vi "single fit V5.vi"(0 "single fit parameters":T11={"number of 2D grid points"=300, "# of points in pond"=339, "# of points in window"=10919, "decimation threshold"=1, "normalization factor"=0.029014793, "pond scale factor "=3.0, "normalized z"=[], "decimated z"=[], "decimated omega"=[], "omega in window"=[], "z in window"=[], "data center"=3.0+0.0i, "inverse"=[], "linear "=[], "omega around"=[], "phase around center"=[], "fit for phase around senter "=[], "three points"={[], []}, "max omega"=0.029014793, "min omega"=0.029014793, "dz/domega"=[]}, 1 "plot what":enum16{"plot", "dont plot", "a"}(ring), 2 "find fit action":T8=enum."bbb", 3 "cursor bracket: fragment  ref":refnum<vi>, 5 "omega map parameters":T10={"map method"=enum."less trivial", "2:window factor"=1, "left"=3.0, "right"=3.0, "omega"=3.0, "gamma"=3.0, "theta0"=3.0, "use points"=enum."decimated", "z(inf) method"=enum."median"}, 7 "parameters: wavepacket":T4={"R"=0.5, "wave number"=9.317073170731707, "delta k"=8.0, "radii vector"=[-1.5, -1.4361702127659575, -1.372340425531915, -1.3085106382978724, -1.2446808510638299, -1.1808510638297873, -1.1170212765957448, -1.0531914893617023, -0.9893617021276596, -0.9255319148936171, -0.8617021276595745, -0.797872340425532, -0.7340425531914894, -0.6702127659574468, -0.6063829787234043, -0.5425531914893618, -0.47872340425531923, -0.4148936170212767, -0.35106382978723416, -0.2872340425531916, -0.2234042553191491, -0.15957446808510656, -0.09574468085106402, -0.03191489361702149, 0.03191489361702127, 0.0957446808510638, 0.15957446808510634, 0.22340425531914887, 0.2872340425531914, 0.35106382978723394, 0.4148936170212765, 0.478723404255319, 0.5425531914893615, 0.6063829787234041, 0.6702127659574466, 0.7340425531914891, 0.7978723404255317, 0.8617021276595742, 0.9255319148936167, 0.9893617021276593, 1.0531914893617018, 1.1170212765957444, 1.1808510638297869, 1.2446808510638294, 1.308510638297872, 1.3723404255319145, 1.436170212765957], "radial section"=[-0.0004435445083409722-0.0006849119769038184i, -0.0019041504025470312+0.00048506615579312746i, -0.00033819317362592454+0.00445256884703147i, 0.008816469374270853+0.0037385059601190047i, 0.012871051762105094-0.014489928742809924i, -0.018368300887416027-0.03213667871181133i, -0.06546452421830008+0.012862287260149104i, -0.014850036489490822+0.11250194158627941i, 0.16349796399613198+0.08029027224632529i, 0.19438455385148304-0.19581588584379236i, -0.1764517694229995-0.3527505964833319i, -0.5269831636950821+0.07349813170268539i, -0.12571385568454752+0.6656158756342778i, 0.7094879059571741+0.3986438774133789i, 0.6853115356988965-0.6177994674685856i, -0.39205198313530026-0.9060192033187687i, -0.9933425353192824+0.08278273424671147i, -0.22770617853759392+0.9220982637950581i, 0.720265950295077+0.4589746661280373i, 0.564369978321562-0.45471185099562045i, -0.20063123992670956-0.5446207511436068i, -0.438459632746935+0.012155082564416607i, -0.0917074180027409+0.299079584121901i, 0.17101533661135507+0.12280738192151135i, 0.17101533661135532+0.1228073819215104i, -0.0917074180027395+0.299079584121901i, -0.4384596327469345+0.01215508256441854i, -0.2006312399267118-0.5446207511436055i, 0.5643699783215596-0.4547118509956226i, 0.7202659502950789+0.45897466612803384i, -0.22770617853759056+0.9220982637950585i, -0.9933425353192818+0.08278273424671675i, -0.3920519831353035-0.9060192033187675i, 0.6853115356988935-0.6177994674685894i, 0.7094879059571758+0.3986438774133766i, -0.12571385568454407+0.665615875634279i, -0.5269831636950825+0.0734981317026883i, -0.17645176942300106-0.3527505964833319i, 0.19438455385148207-0.19581588584379414i, 0.16349796399613292+0.0802902722463243i, -0.014850036489490074+0.11250194158627992i, -0.06546452421830022+0.012862287260149614i, -0.018368300887416446-0.032136678711811265i, 0.012871051762104992-0.014489928742810118i, 0.008816469374270927+0.0037385059601189627i, -0.0003381931736258947+0.004452568847031496i, -0.0019041504025470377+0.00048506615579315077i], "wave vector"=19.513632417419526, "wavepacket is"=TRUE} {"delta k" format="%#_3f"; "wave number" format="%#_3f"; "R" format="%#_3f"}, 9 "parameters: complex fit":T3={"main VI path"=path "", "scale factor"=3.0, "# of grid points"=200, "parameters: wavepacket"={"R"=0.5, "wave number"=22.0, "delta k"=7.0, "radii vector"=[], "radial section"=[], "wave vector"=22.0, "wavepacket is"=TRUE}, "span"=0.27789, "interference ?"=enum."cp z center", "filter method"=enum."three"} {"span" min=0.0 max=0.5 step=1e-05 scale=0.0001..0.5 scale format="%#_5f"; "parameters: wavepacket"."delta k" format="%#_3f"; "parameters: wavepacket"."wave number" format="%#_3f"; "parameters: wavepacket"."R" format="%#_3f"}, 11 "input":cdb, 13 "plots: filter related":T6) -> (4 "single fit parameters out":T11={"number of 2D grid points"=300, "# of points in pond"=339, "# of points in window"=10919, "decimation threshold"=1, "normalization factor"=0.029014793, "pond scale factor "=3.0, "normalized z"=[], "decimated z"=[], "decimated omega"=[], "omega in window"=[], "z in window"=[], "data center"=3.0+0.0i, "inverse"=[], "linear "=[], "omega around"=[], "phase around center"=[], "fit for phase around senter "=[], "three points"={[], []}, "max omega"=0.029014793, "min omega"=0.029014793, "dz/domega"=[]}, 6 "omega map parameters out":T10={"map method"=enum."less trivial", "2:window factor"=1, "left"=3.0, "right"=3.0, "omega"=3.0, "gamma"=3.0, "theta0"=3.0, "use points"=enum."decimated", "z(inf) method"=enum."median"}, 8 "parameters: wavepacket  out":T4={"R"=0.5, "wave number"=9.317073170731707, "delta k"=8.0, "radii vector"=[-1.5, -1.4361702127659575, -1.372340425531915, -1.3085106382978724, -1.2446808510638299, -1.1808510638297873, -1.1170212765957448, -1.0531914893617023, -0.9893617021276596, -0.9255319148936171, -0.8617021276595745, -0.797872340425532, -0.7340425531914894, -0.6702127659574468, -0.6063829787234043, -0.5425531914893618, -0.47872340425531923, -0.4148936170212767, -0.35106382978723416, -0.2872340425531916, -0.2234042553191491, -0.15957446808510656, -0.09574468085106402, -0.03191489361702149, 0.03191489361702127, 0.0957446808510638, 0.15957446808510634, 0.22340425531914887, 0.2872340425531914, 0.35106382978723394, 0.4148936170212765, 0.478723404255319, 0.5425531914893615, 0.6063829787234041, 0.6702127659574466, 0.7340425531914891, 0.7978723404255317, 0.8617021276595742, 0.9255319148936167, 0.9893617021276593, 1.0531914893617018, 1.1170212765957444, 1.1808510638297869, 1.2446808510638294, 1.308510638297872, 1.3723404255319145, 1.436170212765957], "radial section"=[-0.0004435445083409722-0.0006849119769038184i, -0.0019041504025470312+0.00048506615579312746i, -0.00033819317362592454+0.00445256884703147i, 0.008816469374270853+0.0037385059601190047i, 0.012871051762105094-0.014489928742809924i, -0.018368300887416027-0.03213667871181133i, -0.06546452421830008+0.012862287260149104i, -0.014850036489490822+0.11250194158627941i, 0.16349796399613198+0.08029027224632529i, 0.19438455385148304-0.19581588584379236i, -0.1764517694229995-0.3527505964833319i, -0.5269831636950821+0.07349813170268539i, -0.12571385568454752+0.6656158756342778i, 0.7094879059571741+0.3986438774133789i, 0.6853115356988965-0.6177994674685856i, -0.39205198313530026-0.9060192033187687i, -0.9933425353192824+0.08278273424671147i, -0.22770617853759392+0.9220982637950581i, 0.720265950295077+0.4589746661280373i, 0.564369978321562-0.45471185099562045i, -0.20063123992670956-0.5446207511436068i, -0.438459632746935+0.012155082564416607i, -0.0917074180027409+0.299079584121901i, 0.17101533661135507+0.12280738192151135i, 0.17101533661135532+0.1228073819215104i, -0.0917074180027395+0.299079584121901i, -0.4384596327469345+0.01215508256441854i, -0.2006312399267118-0.5446207511436055i, 0.5643699783215596-0.4547118509956226i, 0.7202659502950789+0.45897466612803384i, -0.22770617853759056+0.9220982637950585i, -0.9933425353192818+0.08278273424671675i, -0.3920519831353035-0.9060192033187675i, 0.6853115356988935-0.6177994674685894i, 0.7094879059571758+0.3986438774133766i, -0.12571385568454407+0.665615875634279i, -0.5269831636950825+0.0734981317026883i, -0.17645176942300106-0.3527505964833319i, 0.19438455385148207-0.19581588584379414i, 0.16349796399613292+0.0802902722463243i, -0.014850036489490074+0.11250194158627992i, -0.06546452421830022+0.012862287260149614i, -0.018368300887416446-0.032136678711811265i, 0.012871051762104992-0.014489928742810118i, 0.008816469374270927+0.0037385059601189627i, -0.0003381931736258947+0.004452568847031496i, -0.0019041504025470377+0.00048506615579315077i], "wave vector"=19.513632417419526, "wavepacket is"=TRUE} {"delta k" format="%#_3f"; "wave number" format="%#_3f"; "R" format="%#_3f"}, 14 "complex region out":T7={"max re"=1.1965102077412717, "min re"=-1.8034897922587283, "max im"=1.1920568931854867, "min im"=-1.636084117505164, "delta re"=3.0, "delta im"=2.8281410106906506, "center re"=-0.3034897922587282, "delta  z"=3.0+2.8281410106906506i, "center im"=-0.2220136121598386, "center z"=-0.3034897922587282+2.8281410106906506i, "d im"=0.0, "d re"=0.0, "d z"=0.0+0.0i}, 15 "lorentzian out":T1={"Amplitude"=-1.0311345636926572, "omega(0)"=-1.0311345636926572, "Gamma"=-1.0311345636926572, "phase"=-1.0311345636926572, "Q"=-1.0311345636926572, "Norm  Ampl"=-1.0311345636926572, "z (inf)"=-1.0311345636926572+0.0i, "4corners"={"z (-pi/2)"=-1.0311345636926572+0.5736824521422934i, "z(inf)"=-0.5200164984937075+1.0975277942502903i, "z (pi/2)"=-1.0311345636926572+0.5736824521422934i, "z center"=-0.5136528600391839+0.580046090596817i, "z(0)"=-0.5200164984937075+1.0975277942502903i, "radius"=-1.0311345636926572}} {"z (inf)" format="%#9_9f"; "Q" format="%#9_9f"; "phase" format="%#9_9f"; "Gamma" format="%#9_9f"; "omega(0)" format="%#9_9f"})   [LabVIEW 2015]
uses:
  lorentzian.ctl
  circle corners.ctl
  complex region.ctl
  single fit parameters.ctl
  omega map parameters.ctl
  cursor winow.ctl
  find peak action.ctl
  wavepacket.ctl
  plot refs -- filter related.ctl
  peak -- parameters -- complex fit.ctl
  filter method control.ctl
  stack action -- control.ctl
  cursor window action.ctl
  Q - not nan -- integer.vi
  peak - simple guess at omega.vi
  peak - less simple guess at omega.vi
  peak - fix phase.vi
  peak - fit phase around center - V1.vi
  peak - geometry fit.vi
  find circle corners V3.vi
  peak - phase around center.vi
  peak - linear and inverse maps.vi
  array smart append -- complex.vi
  array smart append -- real.vi
  array - rotate - col.vi
  array - rotate - row.vi
  array -- 2D mean .vi
  tale of three indices.vi
  filter -- window span logic.vi
  linear interp iiii- complex - z-omega - divide.vi
  linear interpolation iiii- complex.vi
  containing bix.vi
  peak -- guess at omega -- dzdomega.vi
  <vilib>/Utility/error.llb/Clear Errors.vi
  <vilib>/Analysis/baseanly.llb/Median.vi
  <vilib>/Analysis/baseanly.llb/Mean.vi
  <vilib>/Analysis/baseanly.llb/Mean (DBL).vi
  <vilib>/Analysis/2dsp.llb/Unwrap Phase.vi
  <vilib>/Analysis/baseanly.llb/A x B.vi
  <vilib>/Analysis/baseanly.llb/Real A x B.vi
  command stack.vi
  tale of three indices -- check state.vi
  linear interp iiii- complex - z-omega.vi
  line -- complex.vi
  peak -- z center from mult phase points.vi
  peak -- estimate for lorentzian.vi
  peak -- fake phase around center.vi
  peak -- four corner circle transformation logic.vi
  <vilib>/Analysis/baseanly.llb/Complex A x B.vi
  circle center from three points.vi
  index from range.vi
  <vilib>/gmath/interp.llb/Interpolate 1D.vi
  peak -- fit function -- arctan.vi
  <vilib>/gmath/NumericalOptimization/Nonlinear Curve Fit.vi
  <vilib>/gmath/NumericalOptimization/Nonlinear Curve Fit LM.vi
  <vilib>/Analysis/6fits.llb/Linear Fit.vi
  <vilib>/Analysis/Matrix/Numeric/Conversions/Array To Matrix.vi
  <vilib>/Analysis/Matrix/Numeric/Conversions/Array To Matrix - CA2.vi
  <vilib>/Analysis/Matrix/Numeric/Multiply/Multiply.vi
  <vilib>/Analysis/Matrix/Numeric/Multiply/Multiply - C,CM.vi
  <vilib>/Analysis/Matrix/Numeric/Add/Add.vi
  <vilib>/Analysis/Matrix/Numeric/Add/Add - CM,CM.vi
  <vilib>/Analysis/Matrix/Numeric/Complex/Complex To Polar.vi
  <vilib>/Analysis/Matrix/Numeric/Complex/Complex To Polar - CM.vi
  <vilib>/Analysis/Matrix/Numeric/Conversions/Array To Matrix - RA2.vi
  <vilib>/Analysis/baseanly.llb/Inverse Matrix.vi
  <vilib>/Analysis/baseanly.llb/Real Inverse Matrix.vi
  array - generate range.vi
panel:
  out "# points in window":dbl
  out "good lorentzian":T1={"Amplitude"=-1.0311345636926572, "omega(0)"=-1.0311345636926572, "Gamma"=-1.0311345636926572, "phase"=-1.0311345636926572, "Q"=-1.0311345636926572, "Norm  Ampl"=-1.0311345636926572, "z (inf)"=-1.0311345636926572+0.0i, "4corners"={"z (-pi/2)"=-1.0311345636926572+0.5736824521422934i, "z(inf)"=-0.5200164984937075+1.0975277942502903i, "z (pi/2)"=-1.0311345636926572+0.5736824521422934i, "z center"=-0.5136528600391839+0.580046090596817i, "z(0)"=-0.5200164984937075+1.0975277942502903i, "radius"=-1.0311345636926572}} {"z (inf)" format="%#9_9f"; "Q" format="%#9_9f"; "phase" format="%#9_9f"; "Gamma" format="%#9_9f"; "omega(0)" format="%#9_9f"}
  out "cp lorentzian":T1={"Amplitude"=-1.0311345636926572, "omega(0)"=-1.0311345636926572, "Gamma"=-1.0311345636926572, "phase"=-1.0311345636926572, "Q"=-1.0311345636926572, "Norm  Ampl"=-1.0311345636926572, "z (inf)"=-1.0311345636926572+0.0i, "4corners"={"z (-pi/2)"=-1.0311345636926572+0.5736824521422934i, "z(inf)"=-0.5200164984937075+1.0975277942502903i, "z (pi/2)"=-1.0311345636926572+0.5736824521422934i, "z center"=-0.5136528600391839+0.580046090596817i, "z(0)"=-0.5200164984937075+1.0975277942502903i, "radius"=-1.0311345636926572}} {"z (inf)" format="%#9_9f"; "Q" format="%#9_9f"; "phase" format="%#9_9f"; "Gamma" format="%#9_9f"; "omega(0)" format="%#9_9f"}
  out "pm lorentzian":T1={"Amplitude"=-1.0311345636926572, "omega(0)"=-1.0311345636926572, "Gamma"=-1.0311345636926572, "phase"=-1.0311345636926572, "Q"=-1.0311345636926572, "Norm  Ampl"=-1.0311345636926572, "z (inf)"=-1.0311345636926572+0.0i, "4corners"={"z (-pi/2)"=-1.0311345636926572+0.5736824521422934i, "z(inf)"=-0.5200164984937075+1.0975277942502903i, "z (pi/2)"=-1.0311345636926572+0.5736824521422934i, "z center"=-0.5136528600391839+0.580046090596817i, "z(0)"=-0.5200164984937075+1.0975277942502903i, "radius"=-1.0311345636926572}} {"z (inf)" format="%#9_9f"; "Q" format="%#9_9f"; "phase" format="%#9_9f"; "Gamma" format="%#9_9f"; "omega(0)" format="%#9_9f"}
  in  "window factor - max":i32=10
  in  "window factor - min":i32=10
  out "bb 2":dbl
  out "directed sigma 2":dbl
  out "right 2":cdb
  out "left 2":cdb
  out "Numeric 2":i32
  in  "averaging -- win 2":dbl=1.3
  in  "averaging -- span 2":dbl=0.2
  in  "averaging -- # points 2":i32=30
  in  "averaging -- # points":i32=30
  in  "averaging -- span":dbl=0.2
  in  "averaging -- win":dbl=1.3
  out "Numeric":i32
  out "left":cdb
  out "right":cdb
  out "directed sigma":dbl
  out "bb":dbl
  in  "complex region":T7={"max re"=1.1965102077412717, "min re"=-1.8034897922587283, "max im"=1.1920568931854867, "min im"=-1.636084117505164, "delta re"=3.0, "delta im"=2.8281410106906506, "center re"=-0.3034897922587282, "delta  z"=3.0+2.8281410106906506i, "center im"=-0.2220136121598386, "center z"=-0.3034897922587282+2.8281410106906506i, "d im"=0.0, "d re"=0.0, "d z"=0.0+0.0i}
  in  "cursor bracket in":T9={"left"=2044.0881763527054, "right "=2126.7657992565055, "center"=2085.4269878046052, "window"=82.67762290380006, "cursors"=[], "relative"=0, "absolute"=0, "fixed vertical offset"=2421.6740576496672, "vertical offset"=2421.6740576496672, "skew"=2421.6740576496672, "default window frac"=2421.6740576496672, "kind"=enum."fancy", "skew.left"=2.0, "skew.right"=0.0, "Plot ref"=refnum, "wing order"=enum."back"}
  in  "factor":dbl=7.0
  in  "pond":cdb[][](array[numeric])
  in  "wave packet":cdb[][](array[numeric])
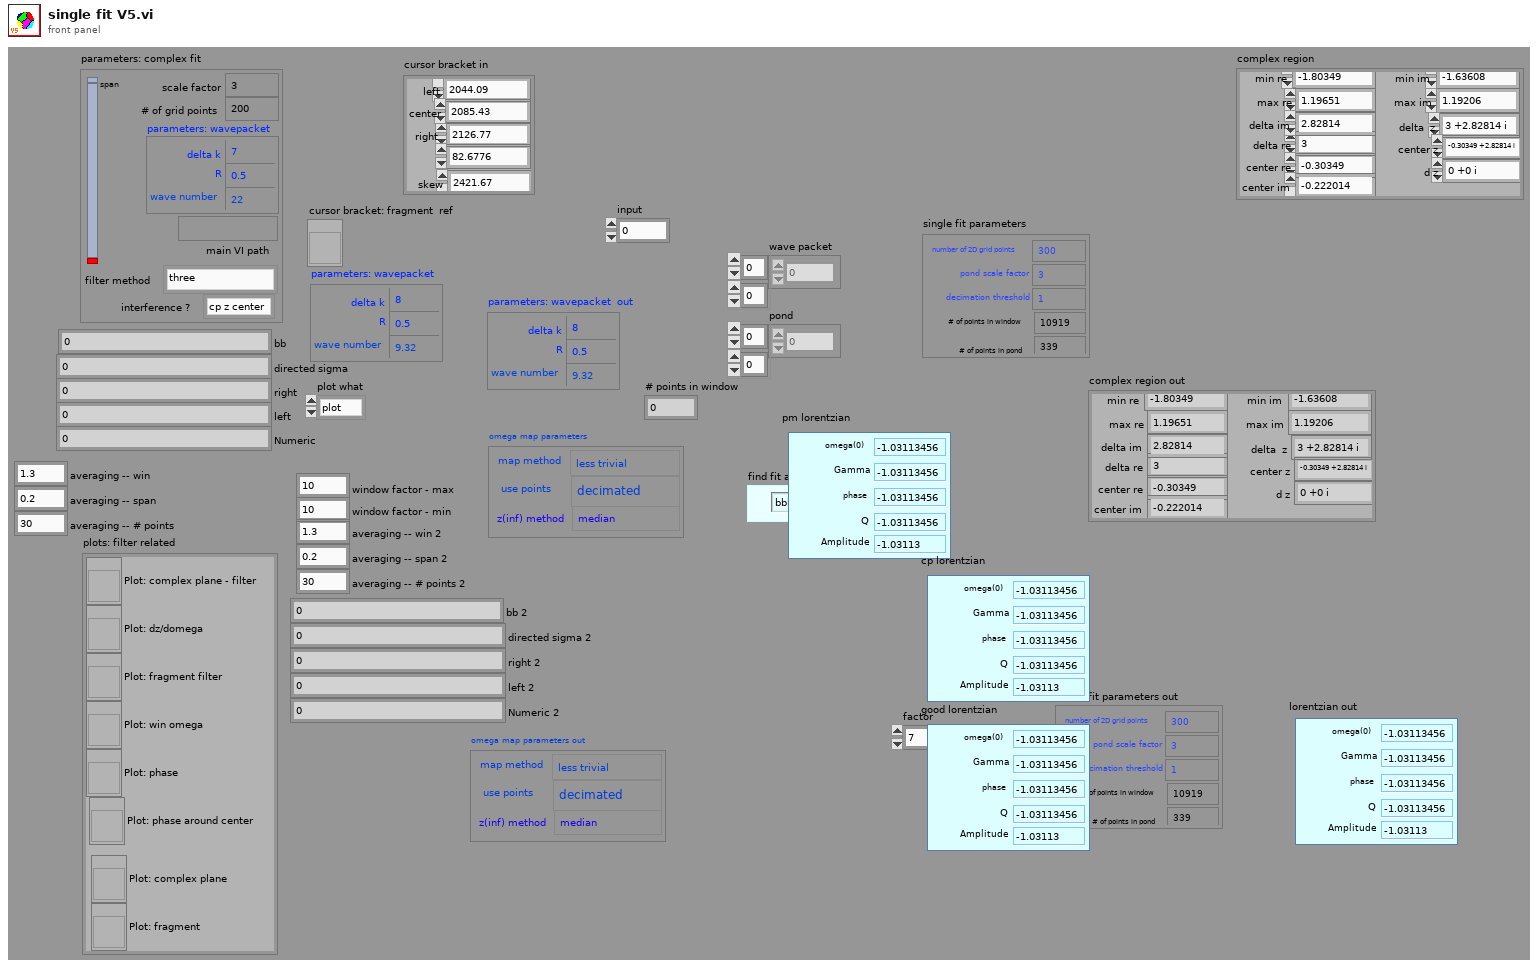
[diagram p1: front panel]
types:
  T1 = typedef "lorentzian.ctl" = cluster{"Amplitude":dbl, "omega(0)":dbl, "Gamma":dbl, "phase":dbl, "Q":dbl, "Norm  Ampl":dbl, "z (inf)":cdb, "4corners":T2}
  T2 = typedef "circle corners.ctl" = cluster{"z (-pi/2)":cdb, "z(inf)":cdb, "z (pi/2)":cdb, "z center":cdb, "z(0)":cdb, "radius":dbl}
  T3 = typedef "peak -- parameters -- complex fit.ctl" = cluster{"main VI path":path, "scale factor":dbl, "# of grid points":i32, "parameters: wavepacket":T4, "span":dbl, "interference ?":enum16{"cp z center", "pm zcenter", "fancy"}, "filter method":T5}
  T4 = typedef "wavepacket.ctl" = cluster{"R":dbl, "wave number":dbl, "delta k":dbl, "radii vector":dbl[], "radial section":cdb[], "wave vector":dbl, "wavepacket is":bool}
  T5 = typedef "filter method control.ctl" = enum16{"four", "five", "one", "two", "three", "zero", "minus one", "minus two"}
  T6 = typedef "plot refs -- filter related.ctl" = cluster{"Plot: complex plane - filter":refnum<vi>, "Plot: dz/domega":refnum<vi>, "Plot: fragment filter":refnum<vi>, "Plot: win omega":refnum<vi>, "Plot: phase":refnum<vi>, "Plot: phase around center":refnum<vi>, "Plot: complex plane":refnum<vi>, "Plot: fragment":refnum<vi>}
  T7 = typedef "complex region.ctl" = cluster{"max re":dbl, "min re":dbl, "max im":dbl, "min im":dbl, "delta re":dbl, "delta im":dbl, "center re":dbl, "delta  z":cdb, "center im":dbl, "center z":cdb, "d im":dbl, "d re":dbl, "d z":cdb}
  T8 = typedef "find peak action.ctl" = enum16{"empty", "-find center", "-mapping", "fit", "-shake it one", "bbb", "-update pond", "move z(center)", "move z(inf)", "update pond", "fancy fit one", "fragment window moves", "-shake it two", "fancy fit two", "pm fit"}
  T9 = typedef "cursor winow.ctl" = cluster{"left":dbl, "right ":dbl, "center":dbl, "window":dbl, "cursors":i32[], "relative":i32, "absolute":i32, "fixed vertical offset":dbl, "vertical offset":dbl, "skew":dbl, "default window frac":dbl, "kind":enum16{"symmetric", "skewed", "fancy"}, "skew.left":dbl, "skew.right":dbl, "Plot ref":refnum<vi>, "wing order":enum16{"forw", "back"}}
  T10 = typedef "omega map parameters.ctl" = cluster{"map method":enum16{"simple", "less trivial", "around center", "geometry"}, "2:window factor":i32, "left":dbl, "right":dbl, "omega":dbl, "gamma":dbl, "theta0":dbl, "use points":enum16{"all in window", "decimated"}, "z(inf) method":enum16{"median", "method 2", "histogram"}}
  T11 = typedef "single fit parameters.ctl" = cluster{"number of 2D grid points":i32, "# of points in pond":i32, "# of points in window":i32, "decimation threshold":i32, "normalization factor":dbl, "pond scale factor ":dbl, "normalized z":cdb[], "decimated z":cdb[], "decimated omega":dbl[], "omega in window":dbl[], "z in window":cdb[], "data center":cdb, "inverse":cdb[], "linear ":cdb[], "omega around":dbl[], "phase around center":dbl[], "fit for phase around senter ":dbl[], "three points":cluster{dbl[], dbl[]}, "max omega":dbl, "min omega":dbl, "dz/domega":cdb[]}
  T12 = cluster{"cursor bracket: fragment  ref":refnum<vi>, "main VI path":path, "fancy fit":cluster{"z(center)":cdb, "center":dbl, "window":dbl, "omega ave":dbl, "gamma ave":dbl, "shakeit counter":i32, "current center":dbl, "current window":dbl}}
  T13 = typedef "stack action -- control.ctl" = enum16{"push", "pop", "check", "init"}
  T14 = typedef "cursor window action.ctl" = enum16{"balance", "h. offset change", "cursor moves", "change center", "change window", "init", "check", "reset", "set y to middle", "idle", "-write all Y", "-write left.X", "-write center.X", "-write right.X", "-write all X", "-change center", "-change window", "-change skew", "-read cursor 2", "-read cursor 1", "-read cursor 0", "-read all cursors", "-reset", "-read plot scale", "-set y to middle", "-Q: center.Y is visible", "-Q: window is visible", "-parse center.Y", "-right left from center", "-left move", "-right move", "-set center.Y", "-empty", "-set cursors to default", "-check", "-write center.Y", "-copy cursor 1", "-copy cursor 0", "-copy cursor 2", "move right", "move left", "shrink", "broaden", "skew up", "skew down", "-write plot scale", "zoom X", "change cen&win", "zoom to all data"}
  T15 = typedef "comparison control.ctl" = enum16{"not a number", "above", "in range", "below"}
  T16 = cluster{"left":dbl, "right ":dbl, "center":dbl, "window":dbl, "cursors":i32[], "relative":i32, "absolute":i32, "fixed vertical offset":dbl, "vertical offset":dbl, "skew":dbl, "default window frac":dbl, "kind":enum16{"symmetric", "skewed", "fancy"}, "skew.left":dbl, "skew.right":dbl, "Plot ref":refnum<vi>, "wing order":enum16{"forw", "back"}}
  T17 = enum16{"replace z(center) -- keepin z(inf) the same", "replace z(inf)  -- keeping z(center) the same"}
  T18 = typedef "tale of three indices -- int -- control.ctl" = cluster{"left":i32, "center":i32, "right":i32, "right most":i32, "left most":i32, "window":i32, "max win factor":i32, "max win":i32, "min win":i32}
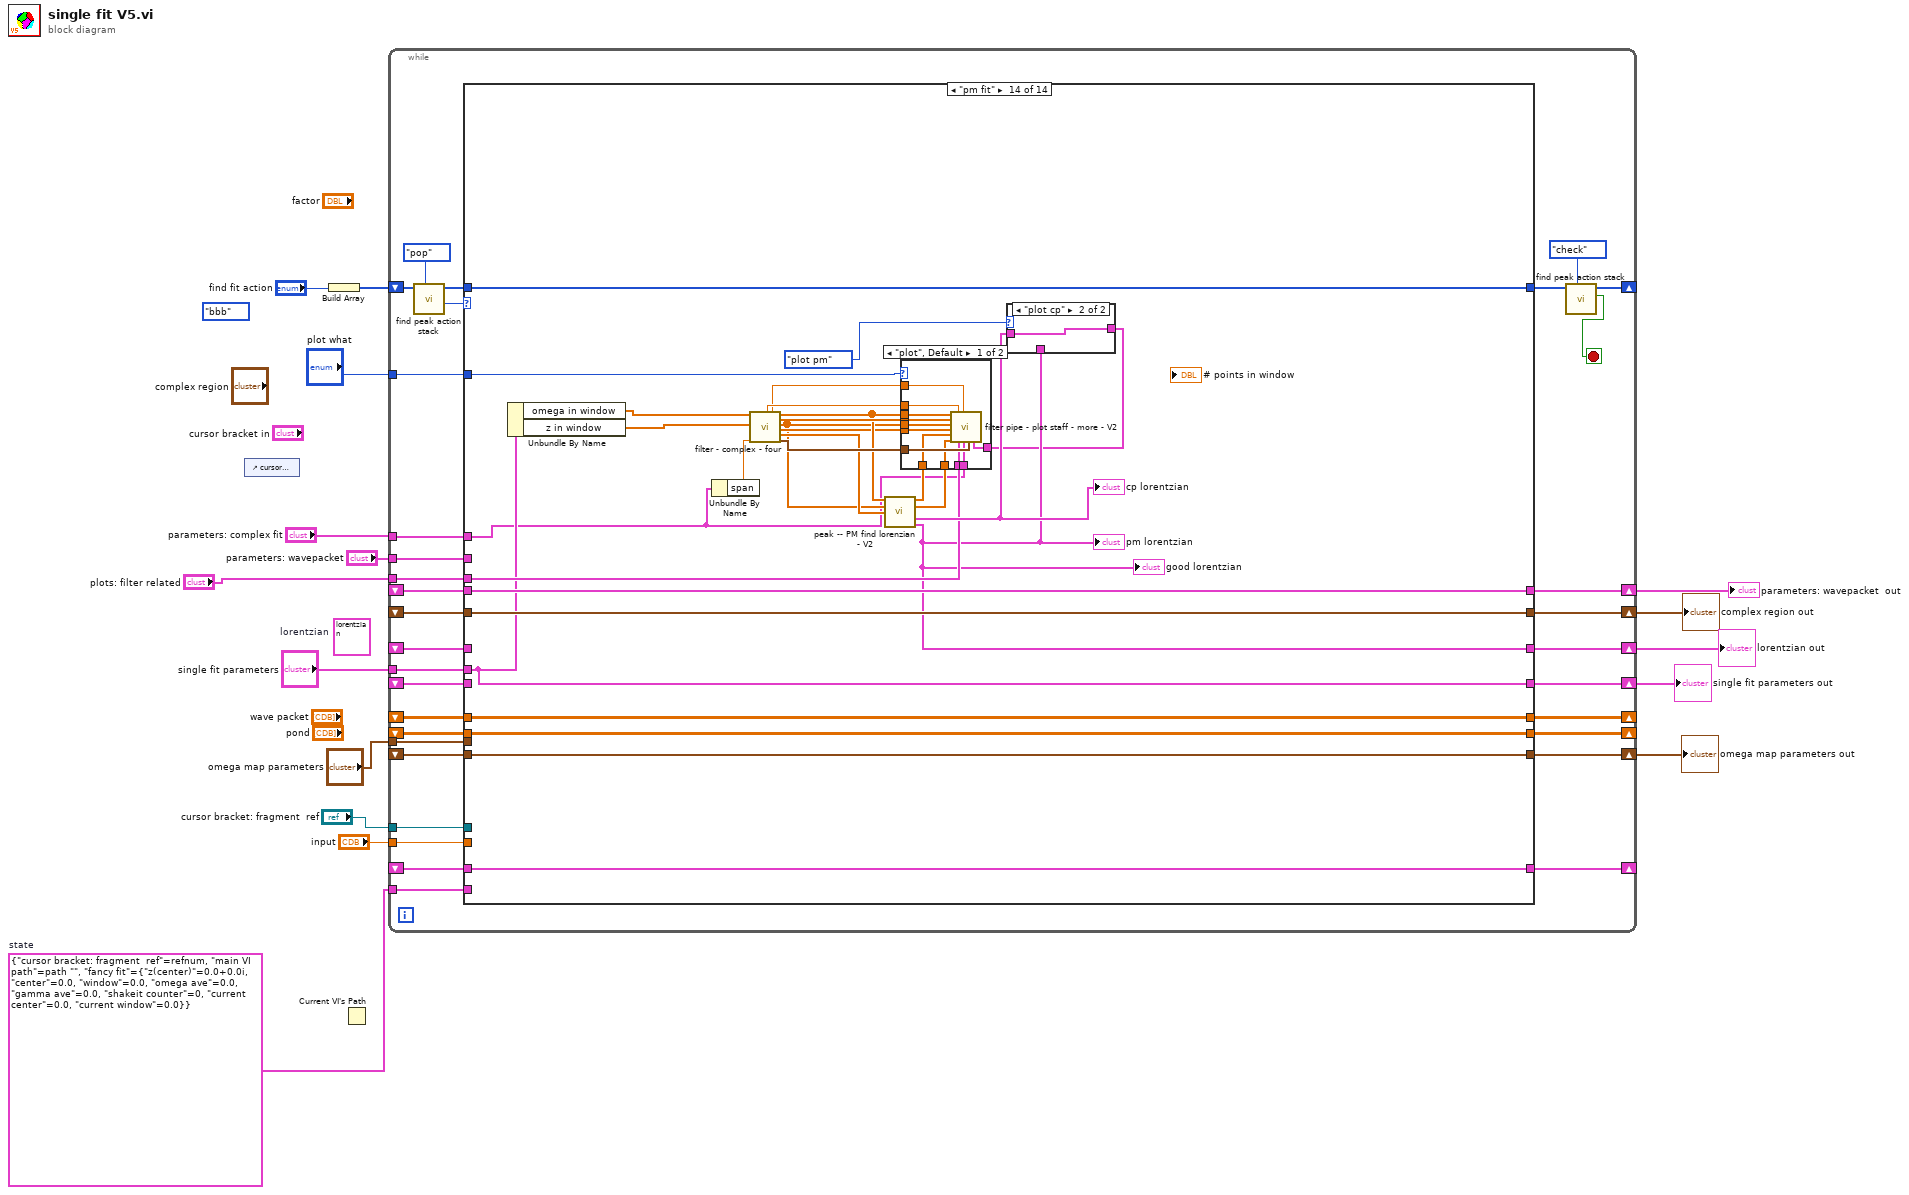
[diagram p0: block diagram]
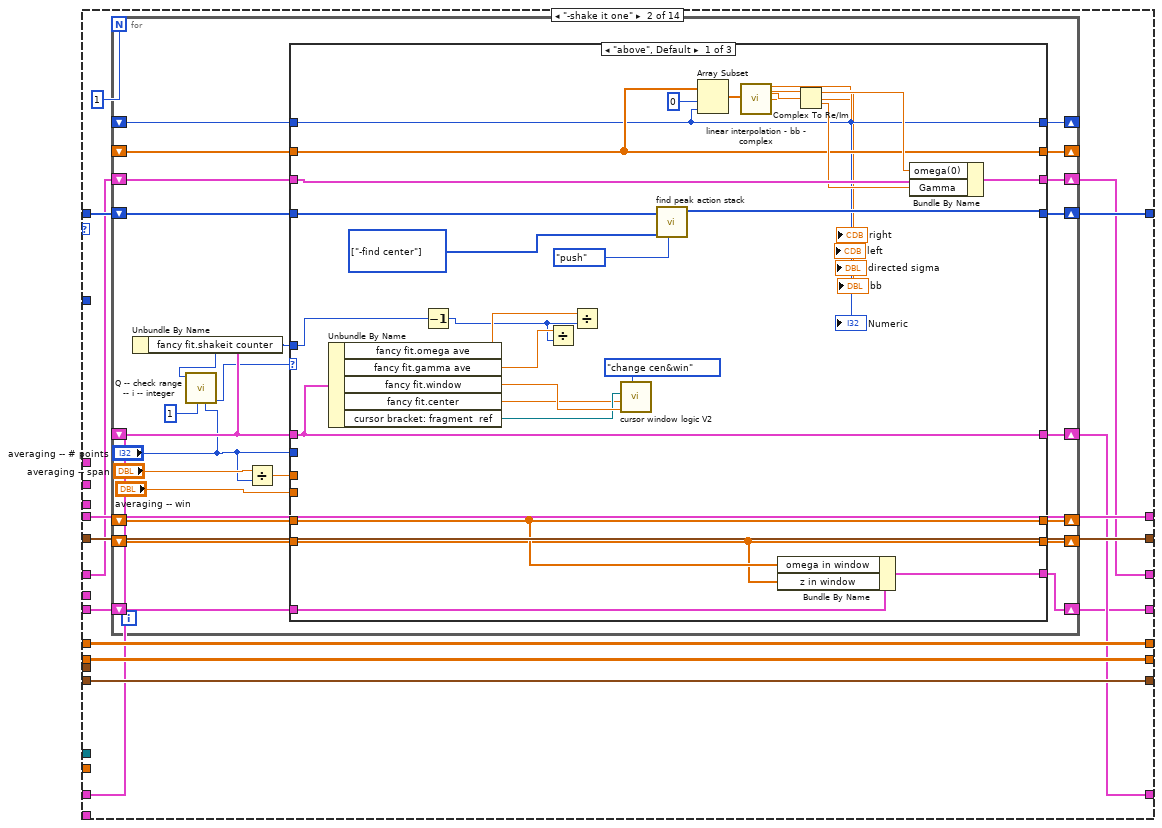
[diagram p3: hidden frame]
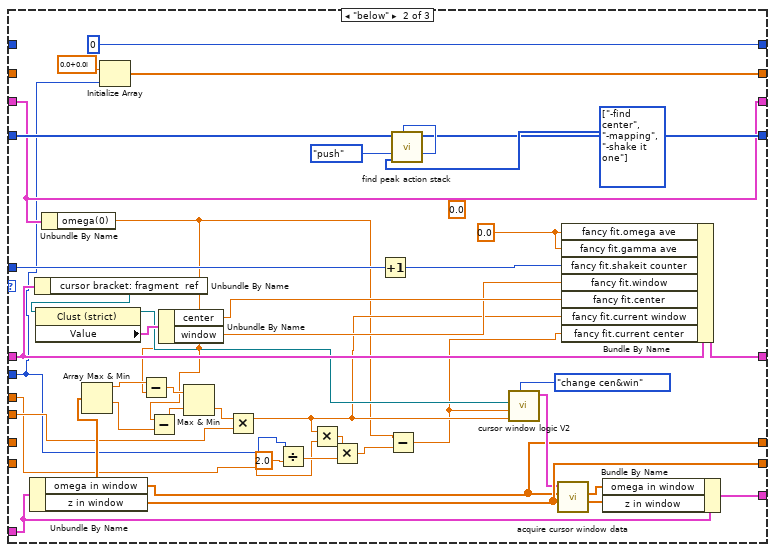
[diagram p4: hidden frame]
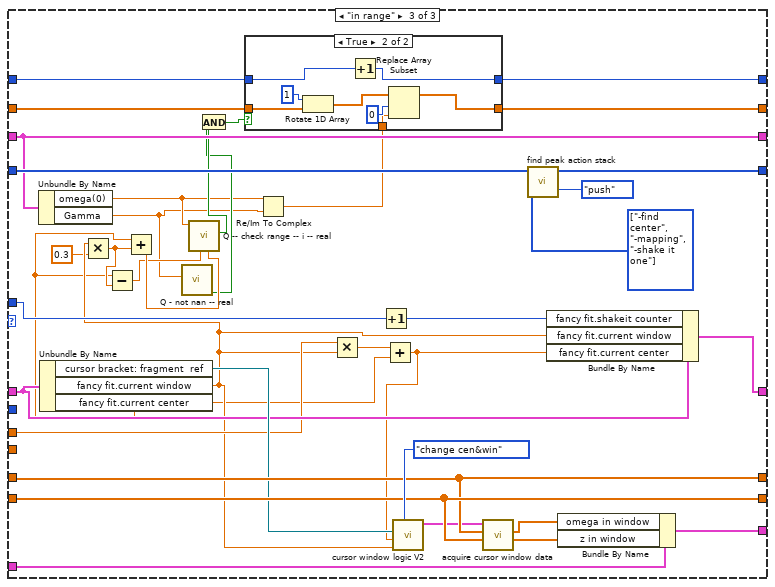
[diagram p5: hidden frame]
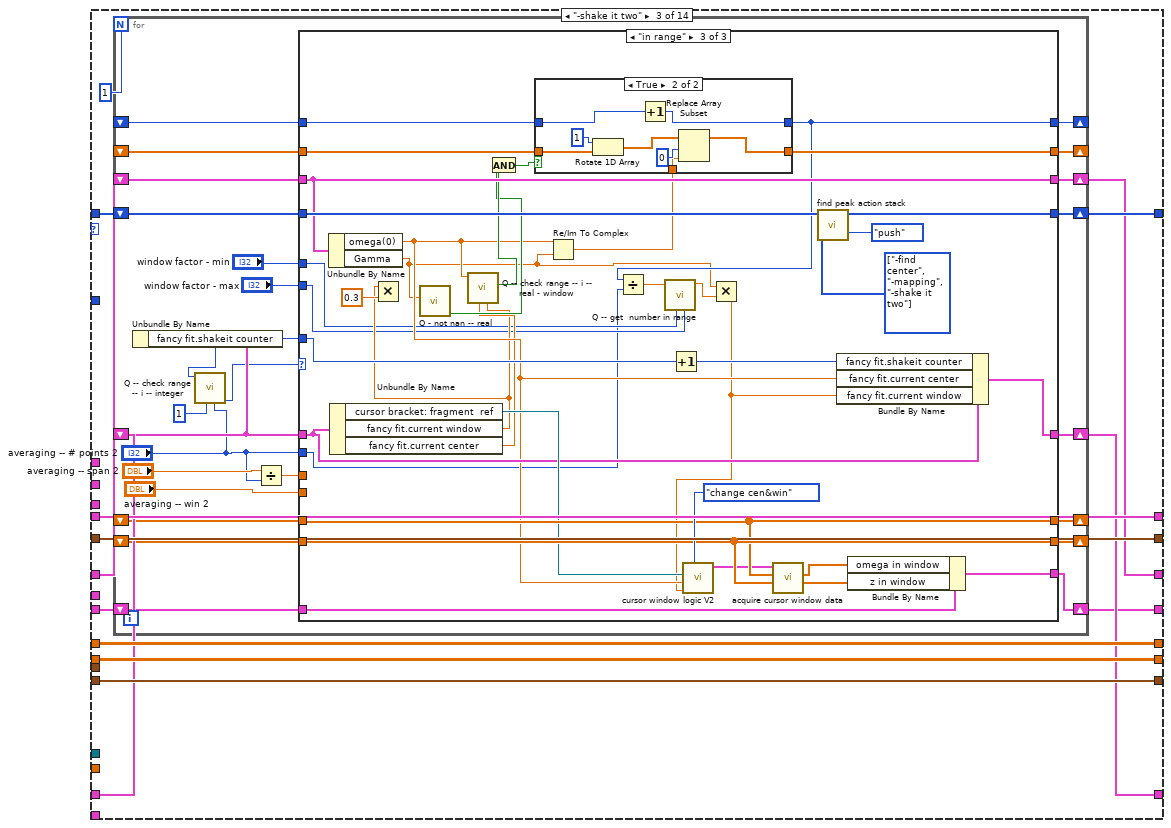
[diagram p7: hidden frame]
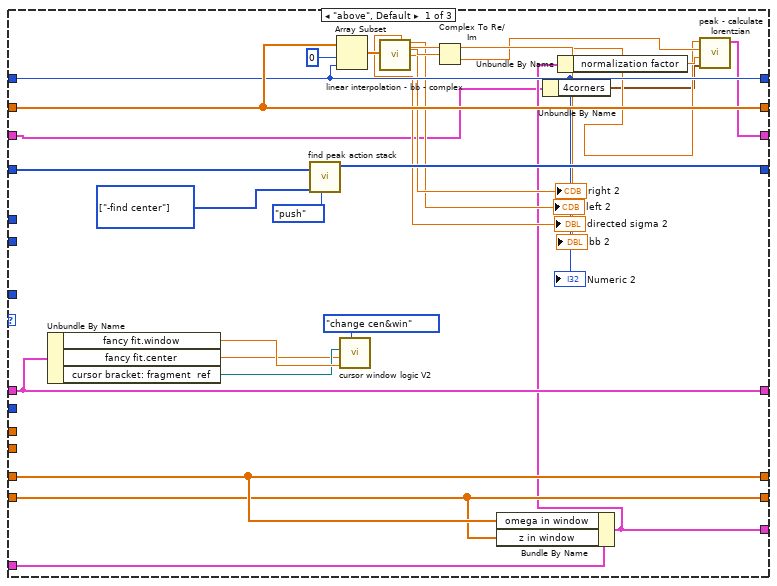
[diagram p8: hidden frame]
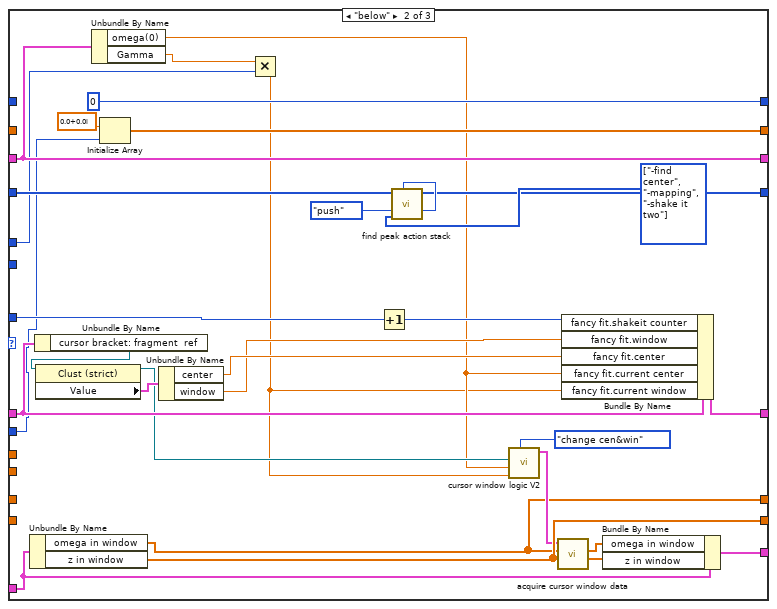
[diagram p9: hidden frame]
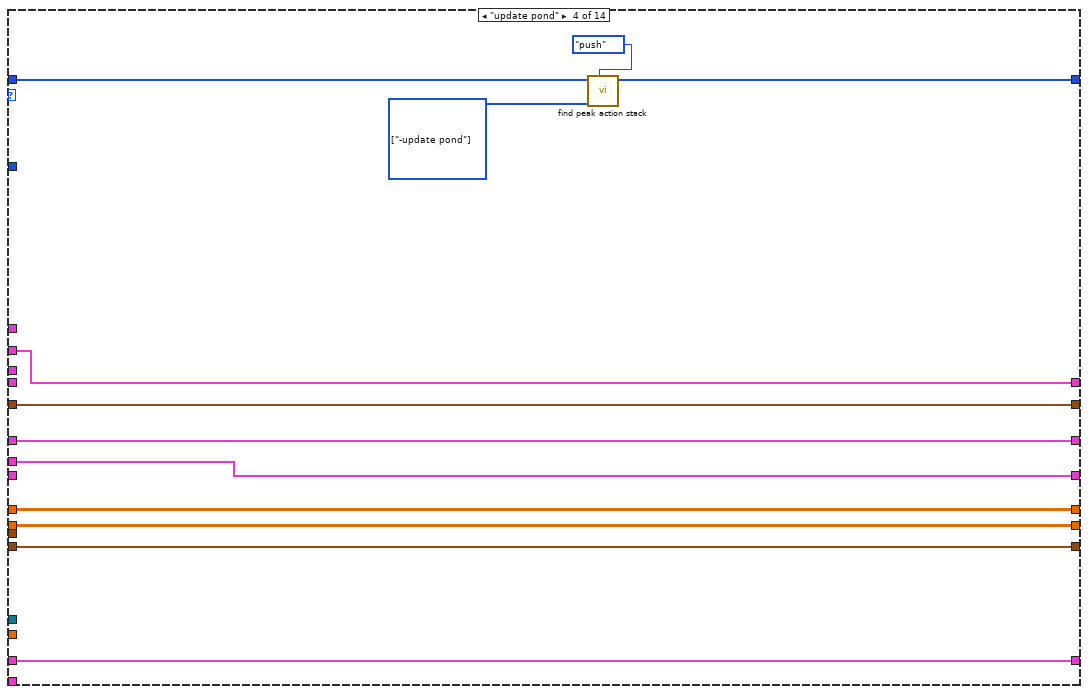
[diagram p11: hidden frame]
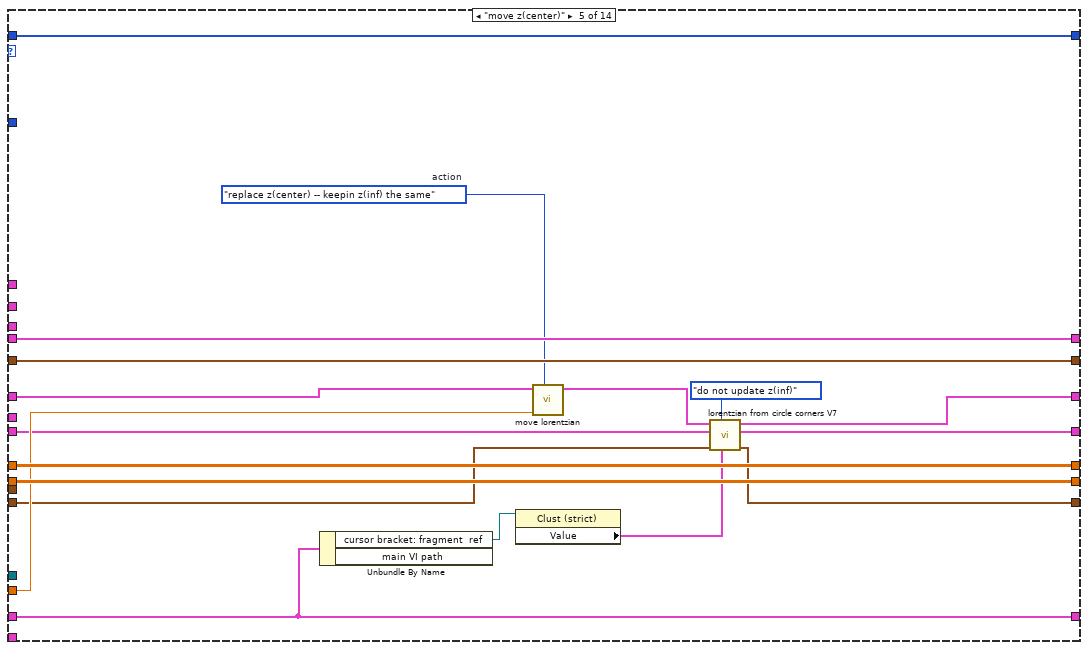
[diagram p12: hidden frame]
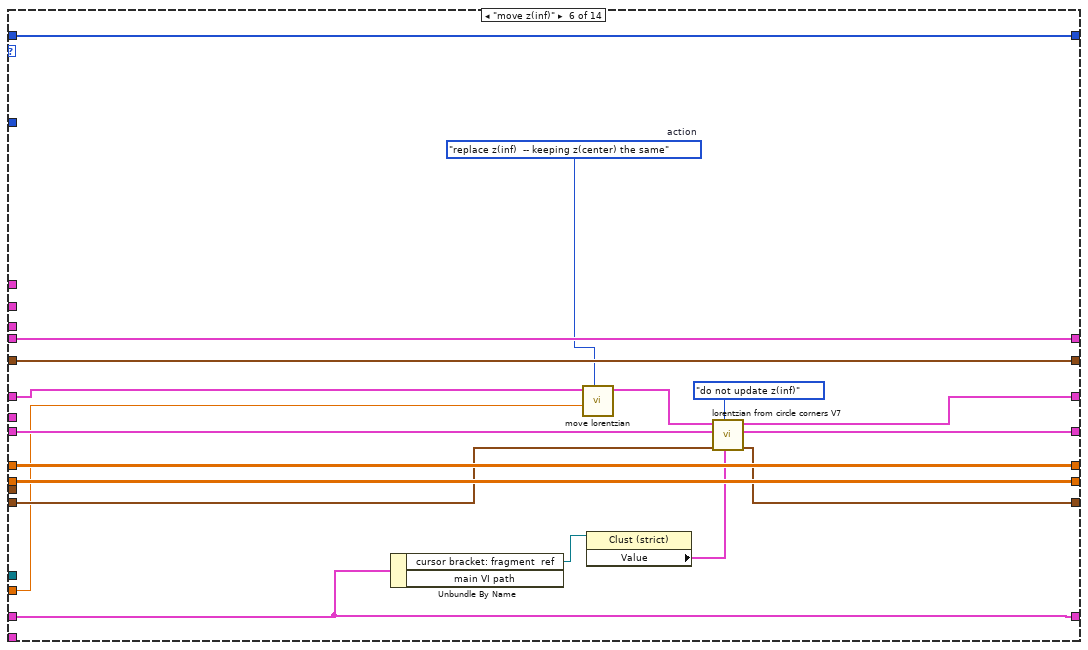
[diagram p13: hidden frame]
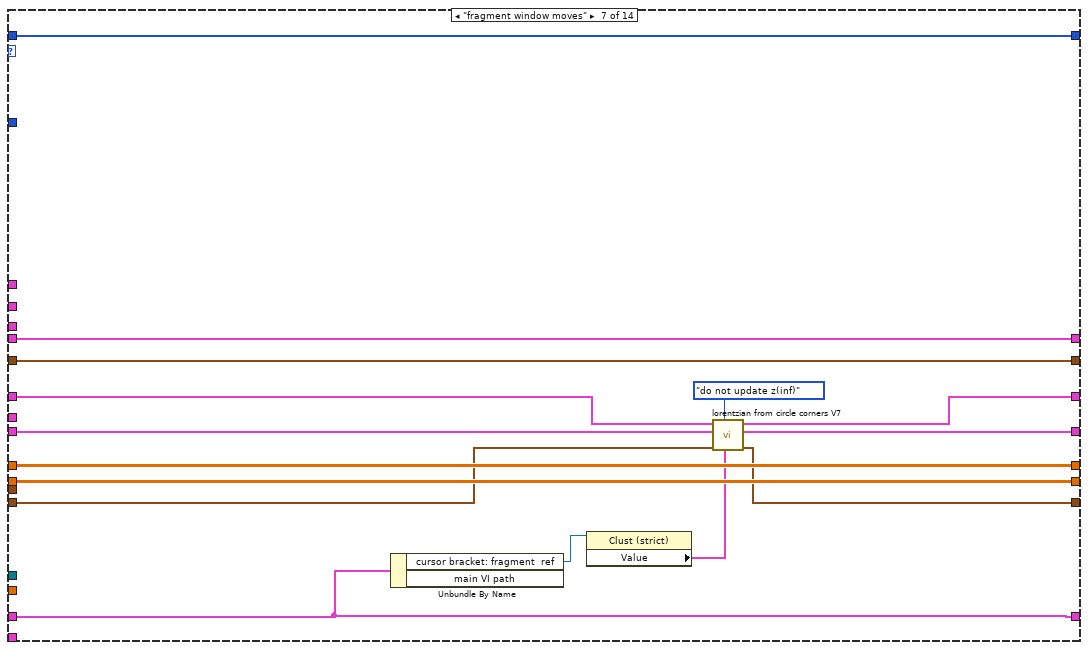
[diagram p14: hidden frame]
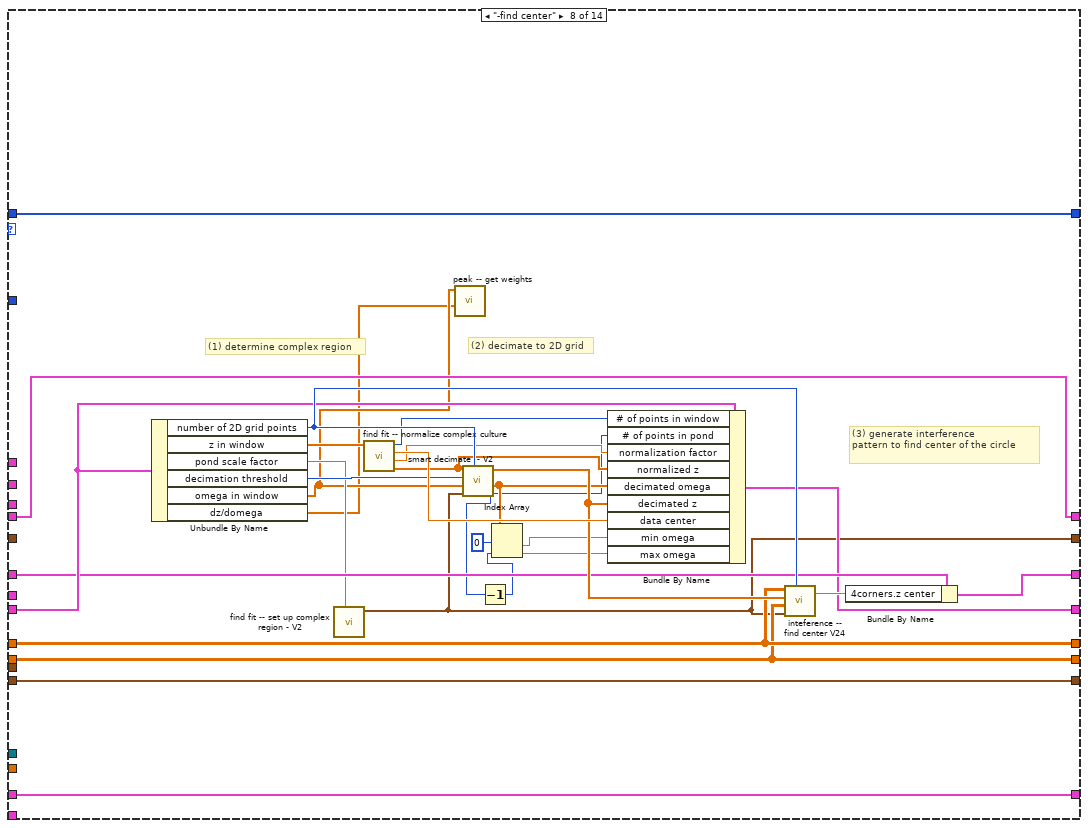
[diagram p15: hidden frame]
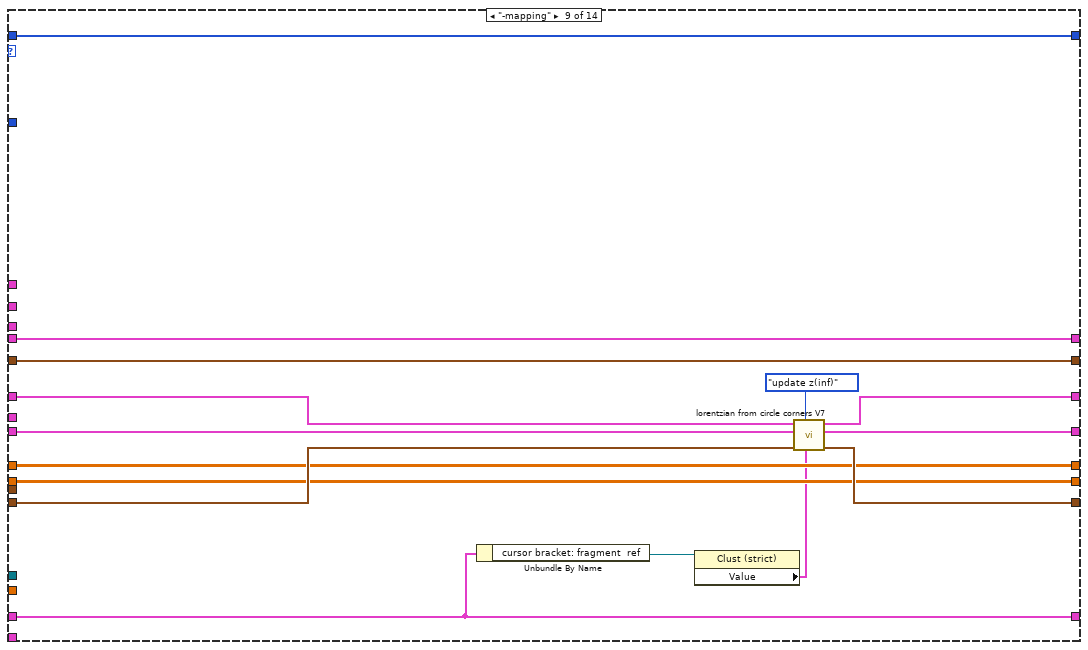
[diagram p16: hidden frame]
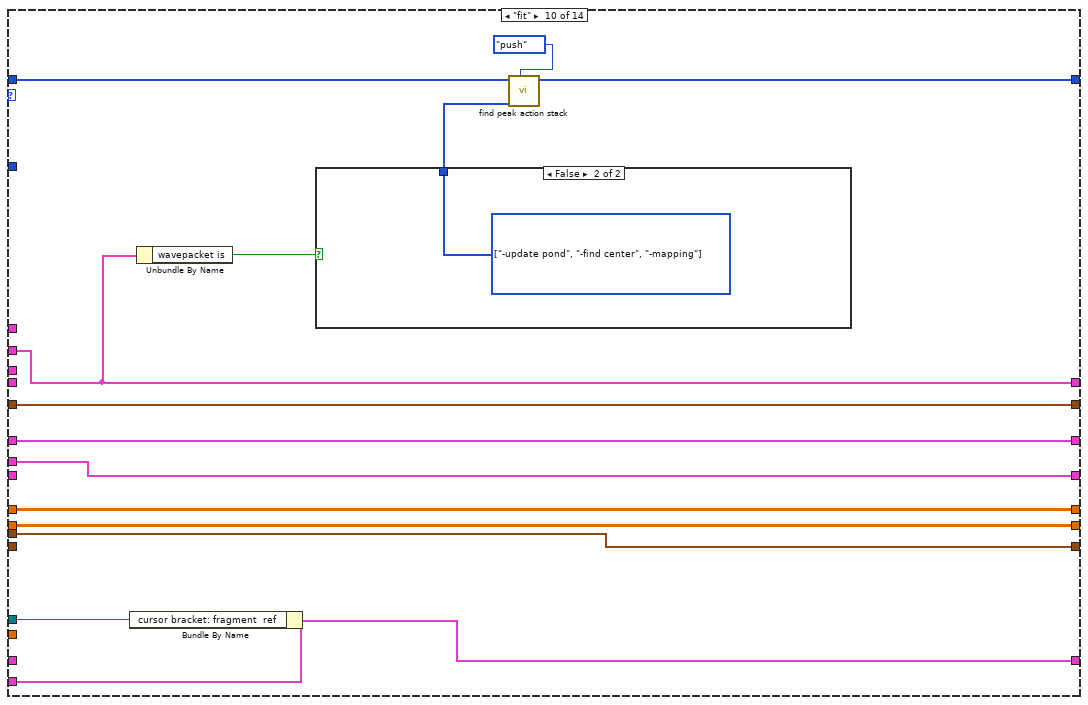
[diagram p17: hidden frame]
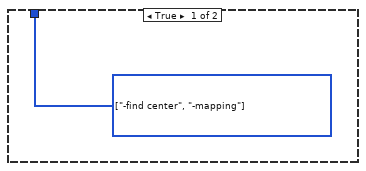
[diagram p18: hidden frame]
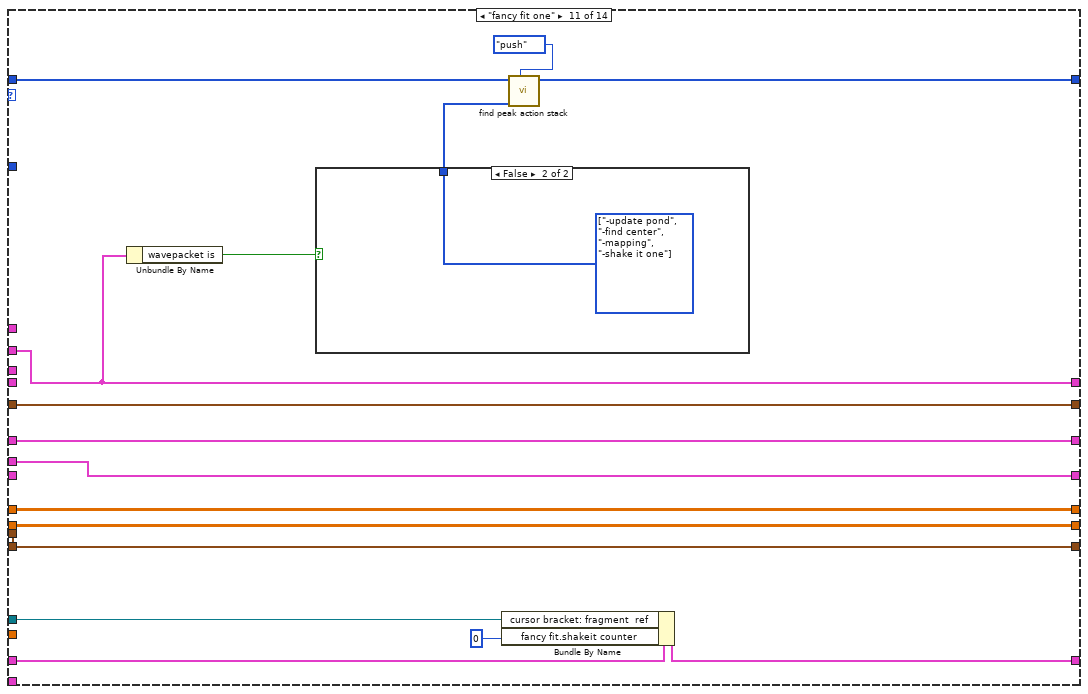
[diagram p19: hidden frame]
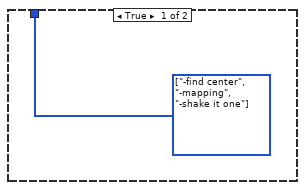
[diagram p20: hidden frame]
diagram:
  w4 = T12 {"cursor bracket: fragment  ref"=refnum, "main VI path"=path "", "fancy fit"={"z(center)"=0.0+0.0i, "center"=0.0, "window"=0.0, "omega ave"=0.0, "gamma ave"=0.0, "shakeit counter"=0, "current center"=0.0, "current window"=0.0}}  # state
  (unwired) find_peak_action."bbb" ("find fit action")
  (unwired) T1 {"Amplitude"=-1.0311345636926572, "omega(0)"=-1.0311345636926572, "Gamma"=-1.0311345636926572, "phase"=-1.0311345636926572, "Q"=-1.0311345636926572, "Norm  Ampl"=-1.0311345636926572, "z (inf)"=-1.0311345636926572+0.0i, "4corners"={"z (-pi/2)"=-1.0311345636926572+0.5736824521422934i, "z(inf)"=-0.5200164984937075+1.0975277942502903i, "z (pi/2)"=-1.0311345636926572+0.5736824521422934i, "z center"=-0.5136528600391839+0.580046090596817i, "z(0)"=-0.5200164984937075+1.0975277942502903i, "radius"=-1.0311345636926572}}  # lorentzian
  n1 = control-ref of="cursor bracket in"() -> ()  [unwired: 1 out]
  n2 = Build Array("find fit action") -> (w15:T8[])
  n3 = Current VI's Path() -> ()  [unwired: 1 out]
  n4 = while {
    shift-right: [w46] -> _
    shift-left: w15 -> [w47]
    shift-right: [w31] -> w12
    shift-left: _ -> [w41]
    shift-right: [w36] -> w13
    shift-left: _ -> [w38]
    shift-right: [w35] -> _
    shift-left: _ -> [w40]
    shift-right: [w34] -> _
    shift-left: _ -> [w39]
    shift-right: [w37] -> w14
    shift-left: _ -> [w30]
    shift-right: [w32] -> w11
    shift-left: _ -> [w33]
    shift-right: [w28] -> w10
    shift-left: _ -> [w29]
    tunnel: "input" -> [w27]
    tunnel: "cursor bracket: fragment  ref" -> [w26]
    tunnel: "single fit parameters" -> [w25]
    tunnel: "omega map parameters" -> [w24]
    tunnel: "parameters: wavepacket" -> [w23]
    shift-right: [w21] -> _
    shift-left: _ -> [w22]
    tunnel: w4 -> [w20]
    tunnel: "plots: filter related" -> [w19]
    tunnel: "parameters: complex fit" -> [w18]
    tunnel: "plot what" -> [w17]
    stop <- w43 stop-if-true
    n5 = call "find peak action stack.vi"("stack action"=stack_action_--_control."pop", "command stack"=w47) -> ("find fit action out"=w42:T8, "command stack out"=w48:T8[])  [unwired: 7 in, 1 out]
    n6 = case shown="\"pm fit\"" w42 {
      tunnel: [w58 w62 w217 w368 w386 w404 w419 w448 w454 w476 w494 w512 w528 w557] -> w49
      tunnel: w48 -> [w58 w67 w222 w368 w386 w404 w419 w448 w454 w478 w496 w514 w528 w557]
      tunnel: w41 -> [w55 w66 w221 _ w375 w394 w411 w439 w459 _ _ _ w521 _]
      tunnel: w40 -> [w53 w70 w225 w364 w384 w402 w417 w436 w456 w472 w490 w508 _ w554]
      tunnel: w39 -> [w52 w69 w224 w363 w383 w401 w416 w435 w455 w471 w489 w507 _ w553]
      tunnel: w38 -> [w56 w63 w218 w366 w373 w392 w405 w438 w460 w473 w491 w509 w530 _]
      tunnel: [w57 w72 w227 w367 w385 w403 w418 w429 w453 w474 w492 w510 w517 w552] -> w37
      tunnel: [w56 w61 w216 w366 w372 w391 w409 w437 w458 w473 w491 w509 w530 w535] -> w36
      tunnel: [w53 w70 w225 w364 w384 w402 w417 w436 w456 w472 w490 w508 w525 w554] -> w35
      tunnel: [w52 w69 w224 w363 w383 w401 w416 w435 w455 w471 w489 w507 w524 w553] -> w34
      tunnel: w33 -> [w54 w71 w226 w365 w377 w396 w413 w433 w462 _ _ _ w529 w558]
      tunnel: [w54 w71 w226 w365 w376 w395 w412 w433 w461 w469 w487 w505 w529 w558] -> w32
      tunnel: [w55 w59 w214 w359 w374 w393 w410 w434 w457 w470 w488 w506 w521 w538] -> w31
      tunnel: w30 -> [w57 w72 w227 w367 w385 w403 w418 _ w453 w474 w492 w510 _ w552]
      tunnel: w29 -> [w51 w68 w223 _ w382 w400 w415 w432 w452 _ _ _ w522 w555]
      tunnel: [w51 w68 w223 w360 w382 w400 w415 w432 w452 w468 w486 w504 w523 w555] -> w28
      tunnel: w27 -> [_ _ _ _ w378 w390 _ _ _ _ _ _ _ _]
      tunnel: w26 -> [_ _ _ _ _ _ _ _ _ w465 w481 w499 _ _]
      tunnel: w25 -> [_ _ _ w359 _ _ _ _ _ w470 w488 w506 _ w538]
      tunnel: w24 -> [_ _ _ _ _ _ _ _ _ w469 w487 w505 _ _]
      tunnel: w23 -> [_ _ _ w360 _ _ _ _ _ w468 w486 w504 _ _]
      tunnel: w22 -> [w50 w64 w219 w358 w370 w387 w406 w431 w450 _ w484 w502 w519 w556]
      tunnel: [w50 w60 w215 w358 w370 w387 w406 w431 w450 w466 w482 w500 w519 w556] -> w21
      tunnel: w20 -> [_ _ _ _ _ _ _ _ _ w464 _ _ _ _]
      tunnel: w19 -> [_ _ _ _ _ _ _ _ _ _ _ _ _ w539]
      tunnel: w18 -> [_ _ _ _ _ _ _ _ _ _ _ _ _ w531]
      tunnel: w17 -> [_ _ _ _ _ _ _ _ _ _ _ _ _ w532]
      frame "empty", Default {
      }
      frame "-shake it one" {
        n7 = for {
          N: 1 -> [_]
          shift-right: [w93] -> _
          shift-left: _ -> [w91]
          shift-right: [w92] -> _
          shift-left: _ -> [w90]
          shift-right: [w87] -> w62
          shift-left: w67 -> [w95]
          shift-right: [w86] -> w61
          shift-left: w63 -> [w88]
          shift-right: [w85] -> w60
          shift-left: w64 -> [w89]
          shift-right: [w84] -> w59
          shift-left: w66 -> [w94]
          shift-right: [w76] -> _
          shift-left: _ -> [w74]
          shift-right: [w75] -> _
          shift-left: _ -> [w73]
          n8 = Unbundle By Name(w89) -> ("fancy fit.shakeit counter"=w81:i32)
          n9 = call "Q -- check range -- i -- integer.vi"("upper"="averaging -- # points", "lower"=1, "number"=w81) -> ("selector"=w82:T15)  [unwired: 6 in, 2 out]
          n10 = Divide(x="averaging -- span", y="averaging -- # points") -> (x/y=w77:dbl)
          n11 = case shown="\"above\", Default" w82 {
            tunnel: w95 -> [w110 w164 w201]
            tunnel: [w109 w163 w200] -> w87
            tunnel: w94 -> [w121 w147 w192]
            tunnel: [w124 w159 w195] -> w84
            tunnel: [w123 w142 w193] -> w93
            tunnel: [w122 w158 w194] -> w92
            tunnel: w91 -> [w123 _ w193]
            tunnel: w90 -> [w122 _ w194]
            tunnel: w89 -> [w114 w153 w189]
            tunnel: [w114 w152 w190] -> w85
            tunnel: w88 -> [w116 w145 w186]
            tunnel: [w115 w145 w186] -> w86
            tunnel: w77 -> [_ w130 w184]
            tunnel: w81 -> [w112 w139 w183]
            tunnel: "averaging -- # points" -> [_ w128 _]
            tunnel: "averaging -- win" -> [_ w131 _]
            tunnel: [w101 w127 w167] -> w76
            tunnel: [w100 0 w172] -> w75
            tunnel: w74 -> [w101 _ w169]
            tunnel: w73 -> [w100 _ w173]
            frame "above", Default {
              w107 = T8[] [enum."-find center"] items=["empty", "-find center", "-mapping", "fit", "-shake it one", "bbb", "-update pond", "move z(center)", "move z(inf)", "update pond", "fancy fit one", "fragment window moves", "-shake it two", "fancy fit two", "pm fit"]
              n12 = Unbundle By Name(w114) -> ("fancy fit.omega ave"=w118:dbl, "fancy fit.gamma ave"=w117:dbl, "fancy fit.window"=w120:dbl, "fancy fit.center"=w113:dbl, "cursor bracket: fragment  ref"=w119:refnum<vi>)
              n13 = Decrement(x=w112) -> (x-1=w111:i32)
              n14 = Divide(x=w117, y=w111) -> ()  [unwired: 1 out]
              n15 = Divide(x=w118, y=w111) -> ()  [unwired: 1 out]
              n16 = call "cursor window logic V2.vi"("cursor window action"=cursor_window_action."change cen&win", "window"=w120, "center"=w113, "cursor window in"=w119) -> ()  [unwired: 6 in, 2 out]
              n17 = call "find peak action stack.vi"("stack action"=stack_action_--_control."push", "find peak action list"=w107, "command stack"=w110) -> ("command stack out"=w109:T8[])  [unwired: 6 in, 2 out]
              n18 = Array Subset(array=w101, index=0, length=w100) -> (w105:cdb[])
              n19 = call "linear interpolation - bb - complex.vi"("Array"=w105) -> ("bb"=→"bb":dbl, "directed sigma"=→"directed sigma":dbl, "left"=→"left":cdb, "center"=w104:cdb, "right"=→"right":cdb)  [unwired: 6 in, 4 out]
              n20 = Bundle By Name(cluster=w121, "omega in window"=w123, "z in window"=w122) -> (w124:T11)
              n21 = Complex To Re/Im(x + iy=w104) -> (x=w103:dbl, y=w102:dbl)
              n22 = Bundle By Name(cluster=w116, "omega(0)"=w103, "Gamma"=w102) -> (w115:T1)
              "Numeric" <- w100
            }
            frame "below" {
              (unwired) 0.0
              w146 = 0.0 ("y")
              w165 = T8[] [enum."-find center", enum."-mapping", enum."-shake it one"] items=["empty", "-find center", "-mapping", "fit", "-shake it one", "bbb", "-update pond", "move z(center)", "move z(inf)", "update pond", "fancy fit one", "fragment window moves", "-shake it two", "fancy fit two", "pm fit"]
              n23 = Unbundle By Name(w147) -> ("omega in window"=w142:dbl[], "z in window"=w158:cdb[])
              n24 = Unbundle By Name(w153) -> ("cursor bracket: fragment  ref"=w150:refnum<vi>)
              n25 = property class="Clust (strict)"(reference=w150) -> (reference out=w143:refnum<vi>, "Value"=w151:T16)  [unwired: 1 in, 1 out]
              n26 = Unbundle By Name(w145) -> ("omega(0)"=w134:dbl)
              n27 = Array Max & Min(array=w142) -> (max value=w141:dbl, min value=w140:dbl)  [unwired: 2 out]
              n28 = Initialize Array(cdb 0.0+0.0i, w128) -> (w127:cdb[])
              n29 = Subtract(x=w141, y=w134) -> (x-y=w155:dbl)
              n30 = Subtract(x=w134, y=w140) -> (x-y=w156:dbl)
              n31 = Unbundle By Name(w151) -> ("center"=w149:dbl, "window"=w148:dbl)
              n32 = Max & Min(x=w155, y=w156) -> (min(x,y)=w157:dbl)  [unwired: 1 out]
              n33 = Multiply(x=w157, y=w131) -> (x*y=w137:dbl)
              n34 = Divide(x=w128, y=2.0) -> (x/y=w135:dbl)
              n35 = Multiply(x=w137, y=w130) -> (x*y=w136:dbl)
              n36 = Multiply(x=w136, y=w135) -> (x*y=w133:dbl)
              n37 = Increment(x=w139) -> (x+1=w154:i32)
              n38 = Subtract(x=w134, y=w133) -> (x-y=w132:dbl)
              n39 = call "find peak action stack.vi"("stack action"=stack_action_--_control."push", "find peak action list"=w165, "command stack"=w164) -> ("command stack out"=w163:T8[])  [unwired: 6 in, 2 out]
              n40 = call "cursor window logic V2.vi"("cursor window action"=cursor_window_action."change cen&win", "window"=w137, "center"=w132, "cursor window in"=w143) -> ("cursor window out"=w144:T9)  [unwired: 6 in, 1 out]
              n41 = call "acquire cursor window data.vi"("z in"=w158, "omega in"=w142, "cursor window"=w144) -> ("z out"=w160:cdb[], "omega  out"=w161:dbl[])  [unwired: 4 in, 3 out]
              n42 = Bundle By Name(cluster=w153, "fancy fit.omega ave"=w146, "fancy fit.gamma ave"=w146, "fancy fit.shakeit counter"=w154, "fancy fit.window"=w148, "fancy fit.center"=w149, "fancy fit.current window"=w137, "fancy fit.current center"=w132) -> (w152:T12)
              n43 = Bundle By Name(cluster=w147, "omega in window"=w161, "z in window"=w160) -> (w159:T11)
            }
            frame "in range" {
              w202 = T8[] [enum."-find center", enum."-mapping", enum."-shake it one"] items=["empty", "-find center", "-mapping", "fit", "-shake it one", "bbb", "-update pond", "move z(center)", "move z(inf)", "update pond", "fancy fit one", "fragment window moves", "-shake it two", "fancy fit two", "pm fit"]
              n44 = Unbundle By Name(w186) -> ("omega(0)"=w171:dbl, "Gamma"=w170:dbl)
              n45 = Unbundle By Name(w189) -> ("cursor bracket: fragment  ref"=w191:refnum<vi>, "fancy fit.current window"=w182:dbl, "fancy fit.current center"=w178:dbl)
              n46 = Multiply(x=w182, y=0.3 ("x")) -> (x*y=w179:dbl)
              n47 = Subtract(x=w178, y=w179) -> (x-y=w177:dbl)
              n48 = Add(x=w178, y=w179) -> (x+y=w180:dbl)
              n49 = call "Q - not nan -- real.vi"("Numeric"=w170) -> ("Boolean"=w175:bool)  [unwired: 9 in, 1 out]
              n50 = call "Q -- check range -- i -- real.vi"("upper"=w180, "lower"=w177, "number"=w171) -> ("in range?"=w176:bool)  [unwired: 6 in, 2 out]
              n51 = And(x=w175, y=w176) -> (x .and. y?=w174:bool)
              n52 = Re/Im To Complex(1:w170, 2:w171) -> (0:w168:cdb)
              n53 = case shown="True" w174 {
                tunnel: w173 -> [w204 w213]
                tunnel: [w204 w212] -> w172
                tunnel: w169 -> [w205 w209]
                tunnel: w168 -> [_ w207]
                tunnel: [w205 w206] -> w167
                frame False {
                }
                frame True {
                  n54 = Rotate 1D Array(1:w209, 2:1) -> (0:w210:cdb[])
                  n55 = Increment(x=w213) -> (x+1=w212:i32)
                  n56 = Replace Array Subset(array=w210, new element=w207, index=0) -> (w206:cdb[])
                }
              }
              n57 = Multiply(x=w184, y=w182) -> (x*y=w199:dbl)
              n58 = Increment(x=w183) -> (x+1=w188:i32)
              n59 = Add(x=w199, y=w178) -> (x+y=w187:dbl)
              n60 = call "cursor window logic V2.vi"("cursor window action"=cursor_window_action."change cen&win", "window"=w182, "center"=w187, "cursor window in"=w191) -> ("cursor window out"=w185:T9)  [unwired: 6 in, 1 out]
              n61 = call "acquire cursor window data.vi"("z in"=w194, "omega in"=w193, "cursor window"=w185) -> ("z out"=w196:cdb[], "omega  out"=w197:dbl[])  [unwired: 4 in, 3 out]
              n62 = call "find peak action stack.vi"("stack action"=stack_action_--_control."push", "find peak action list"=w202, "command stack"=w201) -> ("command stack out"=w200:T8[])  [unwired: 6 in, 2 out]
              n63 = Bundle By Name(cluster=w189, "fancy fit.shakeit counter"=w188, "fancy fit.current window"=w182, "fancy fit.current center"=w187) -> (w190:T12)
              n64 = Bundle By Name(cluster=w192, "omega in window"=w197, "z in window"=w196) -> (w195:T11)
            }
          }
        }
      }
      frame "-shake it two" {
        n65 = for {
          N: 1 -> [_]
          shift-right: [w250] -> _
          shift-left: _ -> [w248]
          shift-right: [w249] -> _
          shift-left: _ -> [w247]
          shift-right: [w244] -> w217
          shift-left: w222 -> [w252]
          shift-right: [w243] -> w216
          shift-left: w218 -> [w245]
          shift-right: [w242] -> w215
          shift-left: w219 -> [w246]
          shift-right: [w241] -> w214
          shift-left: w221 -> [w251]
          shift-right: [w233] -> _
          shift-left: _ -> [w231]
          shift-right: [w232] -> _
          shift-left: _ -> [w230]
          n66 = Unbundle By Name(w246) -> ("fancy fit.shakeit counter"=w238:i32)
          n67 = call "Q -- check range -- i -- integer.vi"("upper"="averaging -- # points 2", "lower"=1, "number"=w238) -> ("selector"=w239:T15)  [unwired: 6 in, 2 out]
          n68 = Divide(x="averaging -- span 2", y="averaging -- # points 2") -> (x/y=w234:dbl)
          n69 = case shown="\"in range\"" w239 {
            tunnel: w252 -> [w273 w308 w345]
            tunnel: [w272 w307 w344] -> w244
            tunnel: w251 -> [w277 w294 w337]
            tunnel: [w258 w303 w340] -> w241
            tunnel: [w279 w290 w338] -> w250
            tunnel: [w278 w302 w339] -> w249
            tunnel: w248 -> [w279 _ w338]
            tunnel: w247 -> [w278 _ w339]
            tunnel: w246 -> [w259 w300 w334]
            tunnel: [w259 w299 w335] -> w242
            tunnel: w245 -> [w255 w293 w332]
            tunnel: [w253 w293 w332] -> w243
            tunnel: w234 -> [_ _ _]
            tunnel: w238 -> [_ w289 w330]
            tunnel: "averaging -- # points 2" -> [_ w287 w314]
            tunnel: "averaging -- win 2" -> [_ _ _]
            tunnel: [w266 w286 w322] -> w233
            tunnel: [w265 0 w315] -> w232
            tunnel: w231 -> [w266 _ w324]
            tunnel: w230 -> [w265 _ w325]
            tunnel: "window factor - min" -> [_ w283 w318]
            tunnel: "window factor - max" -> [_ _ w317]
            frame "above", Default {
              w270 = T8[] [enum."-find center"] items=["empty", "-find center", "-mapping", "fit", "-shake it one", "bbb", "-update pond", "move z(center)", "move z(inf)", "update pond", "fancy fit one", "fragment window moves", "-shake it two", "fancy fit two", "pm fit"]
              n70 = Unbundle By Name(w259) -> ("fancy fit.window"=w276:dbl, "fancy fit.center"=w274:dbl, "cursor bracket: fragment  ref"=w275:refnum<vi>)
              n71 = call "find peak action stack.vi"("stack action"=stack_action_--_control."push", "find peak action list"=w270, "command stack"=w273) -> ("command stack out"=w272:T8[])  [unwired: 6 in, 2 out]
              n72 = Array Subset(array=w266, index=0, length=w265) -> (w268:cdb[])
              n73 = call "cursor window logic V2.vi"("cursor window action"=cursor_window_action."change cen&win", "window"=w276, "center"=w274, "cursor window in"=w275) -> ()  [unwired: 6 in, 2 out]
              n74 = call "linear interpolation - bb - complex.vi"("Array"=w268) -> ("bb"=→"bb 2":dbl, "directed sigma"=→"directed sigma 2":dbl, "left"=→"left 2":cdb, "center"=w267:cdb, "right"=→"right 2":cdb)  [unwired: 6 in, 4 out]
              n75 = Complex To Re/Im(x + iy=w267) -> (x=w256:dbl, y=w257:dbl)
              n76 = Bundle By Name(cluster=w277, "omega in window"=w279, "z in window"=w278) -> (w258:T11)
              n77 = Unbundle By Name(w255) -> ("4corners"=w254:T2)
              n78 = Unbundle By Name(w258) -> ("normalization factor"=w260:dbl)
              n79 = call "peak - calculate lorentzian.vi"("4corners"=w254, "normalization factor"=w260, "gamma"=w257, "omega"=w256) -> ("lorentzian out"=w253:T1)  [unwired: 7 in]
              "Numeric 2" <- w265
            }
            frame "below" {
              w309 = T8[] [enum."-find center", enum."-mapping", enum."-shake it two"] items=["empty", "-find center", "-mapping", "fit", "-shake it one", "bbb", "-update pond", "move z(center)", "move z(inf)", "update pond", "fancy fit one", "fragment window moves", "-shake it two", "fancy fit two", "pm fit"]
              n80 = Unbundle By Name(w294) -> ("omega in window"=w290:dbl[], "z in window"=w302:cdb[])
              n81 = Unbundle By Name(w300) -> ("cursor bracket: fragment  ref"=w297:refnum<vi>)
              n82 = property class="Clust (strict)"(reference=w297) -> (reference out=w291:refnum<vi>, "Value"=w298:T16)  [unwired: 1 in, 1 out]
              n83 = Unbundle By Name(w293) -> ("omega(0)"=w282:dbl, "Gamma"=w284:dbl)
              n84 = Initialize Array(cdb 0.0+0.0i, w287) -> (w286:cdb[])
              n85 = Unbundle By Name(w298) -> ("center"=w296:dbl, "window"=w295:dbl)
              n86 = Multiply(x=w284, y=w283) -> (x*y=w281:dbl)
              n87 = Increment(x=w289) -> (x+1=w301:i32)
              n88 = call "find peak action stack.vi"("stack action"=stack_action_--_control."push", "find peak action list"=w309, "command stack"=w308) -> ("command stack out"=w307:T8[])  [unwired: 6 in, 2 out]
              n89 = call "cursor window logic V2.vi"("cursor window action"=cursor_window_action."change cen&win", "window"=w281, "center"=w282, "cursor window in"=w291) -> ("cursor window out"=w292:T9)  [unwired: 6 in, 1 out]
              n90 = call "acquire cursor window data.vi"("z in"=w302, "omega in"=w290, "cursor window"=w292) -> ("z out"=w304:cdb[], "omega  out"=w305:dbl[])  [unwired: 4 in, 3 out]
              n91 = Bundle By Name(cluster=w300, "fancy fit.shakeit counter"=w301, "fancy fit.window"=w295, "fancy fit.center"=w296, "fancy fit.current center"=w282, "fancy fit.current window"=w281) -> (w299:T12)
              n92 = Bundle By Name(cluster=w294, "omega in window"=w305, "z in window"=w304) -> (w303:T11)
            }
            frame "in range" {
              w346 = T8[] [enum."-find center", enum."-mapping", enum."-shake it two"] items=["empty", "-find center", "-mapping", "fit", "-shake it one", "bbb", "-update pond", "move z(center)", "move z(inf)", "update pond", "fancy fit one", "fragment window moves", "-shake it two", "fancy fit two", "pm fit"]
              n93 = Unbundle By Name(w332) -> ("omega(0)"=w321:dbl, "Gamma"=w312:dbl)
              n94 = Unbundle By Name(w334) -> ("cursor bracket: fragment  ref"=w336:refnum<vi>, "fancy fit.current window"=w319:dbl, "fancy fit.current center"=w320:dbl)
              n95 = Multiply(x=w319, y=0.3 ("x")) -> ()  [unwired: 1 out]
              n96 = call "Q - not nan -- real.vi"("Numeric"=w312) -> ("Boolean"=w327:bool)  [unwired: 9 in, 1 out]
              n97 = call "Q -- check range -- i -- real - window.vi"("window"=w319, "center"=w320, "number"=w321) -> ("in range?"=w328:bool)  [unwired: 6 in, 2 out]
              n98 = And(x=w327, y=w328) -> (x .and. y?=w326:bool)
              n99 = Re/Im To Complex(1:w312, 2:w321) -> (0:w323:cdb)
              n100 = case shown="True" w326 {
                tunnel: w325 -> [w348 w357]
                tunnel: [w348 w356] -> w315
                tunnel: w324 -> [w349 w353]
                tunnel: w323 -> [_ w351]
                tunnel: [w349 w350] -> w322
                frame False {
                }
                frame True {
                  n101 = Rotate 1D Array(1:w353, 2:1) -> (0:w354:cdb[])
                  n102 = Increment(x=w357) -> (x+1=w356:i32)
                  n103 = Replace Array Subset(array=w354, new element=w351, index=0) -> (w350:cdb[])
                }
              }
              n104 = Divide(x=w315, y=w314) -> (x/y=w316:dbl)
              n105 = call "Q -- get  number in range.vi"("right"=w317, "left"=w318, "fraction"=w316) -> ("number in range"=w313:dbl)  [unwired: 8 in]
              n106 = Increment(x=w330) -> (x+1=w333:i32)
              n107 = Multiply(x=w312, y=w313) -> (x*y=w311:dbl)
              n108 = call "cursor window logic V2.vi"("cursor window action"=cursor_window_action."change cen&win", "window"=w311, "center"=w321, "cursor window in"=w336) -> ("cursor window out"=w331:T9)  [unwired: 6 in, 1 out]
              n109 = call "acquire cursor window data.vi"("z in"=w339, "omega in"=w338, "cursor window"=w331) -> ("z out"=w341:cdb[], "omega  out"=w342:dbl[])  [unwired: 4 in, 3 out]
              n110 = call "find peak action stack.vi"("stack action"=stack_action_--_control."push", "find peak action list"=w346, "command stack"=w345) -> ("command stack out"=w344:T8[])  [unwired: 6 in, 2 out]
              n111 = Bundle By Name(cluster=w334, "fancy fit.shakeit counter"=w333, "fancy fit.current center"=w321, "fancy fit.current window"=w311) -> (w335:T12)
              n112 = Bundle By Name(cluster=w337, "omega in window"=w342, "z in window"=w341) -> (w340:T11)
            }
          }
        }
      }
      frame "update pond" {
        w361 = T8[] [enum."-update pond"] items=["empty", "-find center", "-mapping", "fit", "-shake it one", "bbb", "-update pond", "move z(center)", "move z(inf)", "update pond", "fancy fit one", "fragment window moves", "-shake it two", "fancy fit two", "pm fit"]
        n113 = call "find peak action stack.vi"("stack action"=stack_action_--_control."push", "find peak action list"=w361) -> ()  [unwired: 7 in, 3 out]
      }
      frame "move z(center)" {
        w379 = T17."replace z(center) -- keepin z(inf) the same"  # action
        n114 = Unbundle By Name(w370) -> ("cursor bracket: fragment  ref"=w369:refnum<vi>)  [unwired: 1 out]
        n115 = property class="Clust (strict)"(reference=w369) -> ("Value"=w371:T16)  [unwired: 1 in, 2 out]
        n116 = call "move lorentzian.vi"("action"=w379, "new z(center)"=w378, "lorentzian in"=w373) -> ("lorentzian out"=w380:T1)  [unwired: 8 in]
        n117 = call "lorentzian from circle corners V7.vi"("cursor bracket in"=w371, "update z(inf)"=enum16{"update z(inf)", "do not update z(inf)"}."do not update z(inf)", "omega map rameters in"=w377, "parameters in: center detection"=w375, "lorentzian in"=w380) -> ("omega map parameters  out"=w376:T10, "parameters out  : center detection"=w374:T11, "lorentzian out"=w372:T1)  [unwired: 4 in]
      }
      frame "move z(inf)" {
        w397 = T17."replace z(inf)  -- keeping z(center) the same"  # action
        n118 = Unbundle By Name(w387) -> ("cursor bracket: fragment  ref"=w389:refnum<vi>)  [unwired: 1 out]
        n119 = call "move lorentzian.vi"("action"=w397, "new z(inf)"=w390, "lorentzian in"=w392) -> ("lorentzian out"=w398:T1)  [unwired: 8 in]
        n120 = property class="Clust (strict)"(reference=w389) -> ("Value"=w388:T16)  [unwired: 1 in, 2 out]
        n121 = call "lorentzian from circle corners V7.vi"("cursor bracket in"=w388, "update z(inf)"=enum16{"update z(inf)", "do not update z(inf)"}."do not update z(inf)", "omega map rameters in"=w396, "parameters in: center detection"=w394, "lorentzian in"=w398) -> ("omega map parameters  out"=w395:T10, "parameters out  : center detection"=w393:T11, "lorentzian out"=w391:T1)  [unwired: 4 in]
      }
      frame "fragment window moves" {
        n122 = Unbundle By Name(w406) -> ("cursor bracket: fragment  ref"=w408:refnum<vi>)  [unwired: 1 out]
        n123 = property class="Clust (strict)"(reference=w408) -> ("Value"=w407:T16)  [unwired: 1 in, 2 out]
        n124 = call "lorentzian from circle corners V7.vi"("cursor bracket in"=w407, "update z(inf)"=enum16{"update z(inf)", "do not update z(inf)"}."do not update z(inf)", "omega map rameters in"=w413, "parameters in: center detection"=w411, "lorentzian in"=w405) -> ("omega map parameters  out"=w412:T10, "parameters out  : center detection"=w410:T11, "lorentzian out"=w409:T1)  [unwired: 4 in]
      }
      frame "-find center" {
        # "(1) determine complex region"
        # "(3) generate interference\npattern to find center of the circle"
        # "(2) decimate to 2D grid"
        n125 = Unbundle By Name(w439) -> ("number of 2D grid points"=w446:i32, "z in window"=w447:cdb[], "pond scale factor"=w430:dbl, "decimation threshold"=w440:i32, "omega in window"=w421:dbl[], "dz/domega"=w420:cdb[])
        n126 = call "find fit -- set up complex region - V2.vi"("scale factor"=w430) -> ("complex region"=w429:T7)  [unwired: 10 in]
        n127 = call "find fit -- normalize complex culture.vi"("z in window"=w447) -> ("z  normalized"=w442:cdb[], "normalization factor"=w443:dbl, "data center"=w444:cdb, "# of elements"=w426:i32)  [unwired: 7 in]
        n128 = call "peak -- get weights.vi"("dz/domega"=w420, "omega"=w421) -> ()  [unwired: 8 in, 2 out]
        n129 = call "smart decimate  - V2.vi"("number of 2D grid points"=w446, "complex region"=w429, "omega in"=w421, "decimation threshold"=w440, "z in"=w442) -> ("number of decimated elements"=w425:i32, "decimated omega"=w428:dbl[], "decimated z"=w441:cdb[])  [unwired: 4 in]
        n130 = Decrement(x=w425) -> (x-1=w424:i32)
        n131 = Index Array(array=w428, index #1=0 ("index"), index #2=w424) -> (element #1=w423:dbl, element #2=w422:dbl)
        n132 = Bundle By Name(cluster=w439, "# of points in window"=w426, "# of points in pond"=w425, "normalization factor"=w443, "normalized z"=w442, "decimated omega"=w428, "decimated z"=w441, "data center"=w444, "min omega"=w423, "max omega"=w422) -> (w434:T11)
        n133 = call "inteference -- find center V24.vi"("number of points"=w446, "complex region"=w429, "pond"=w435, "point sources"=w441, "wave packet"=w436) -> ("z (center)"=w445:cdb)  [unwired: 6 in]
        n134 = Bundle By Name(cluster=w438, "4corners.z center"=w445) -> (w437:T1)
      }
      frame "-mapping" {
        n135 = Unbundle By Name(w450) -> ("cursor bracket: fragment  ref"=w451:refnum<vi>)
        n136 = property class="Clust (strict)"(reference=w451) -> ("Value"=w449:T16)  [unwired: 1 in, 2 out]
        n137 = call "lorentzian from circle corners V7.vi"("cursor bracket in"=w449, "update z(inf)"=enum16{"update z(inf)", "do not update z(inf)"}."update z(inf)", "omega map rameters in"=w462, "parameters in: center detection"=w459, "lorentzian in"=w460) -> ("omega map parameters  out"=w461:T10, "parameters out  : center detection"=w457:T11, "lorentzian out"=w458:T1)  [unwired: 4 in]
      }
      frame "fit" {
        n138 = Bundle By Name(cluster=w464, "cursor bracket: fragment  ref"=w465) -> (w466:T12)
        n139 = Unbundle By Name(w468) -> ("wavepacket is"=w467:bool)
        n140 = case shown="False" w467 {
          tunnel: [w479 w480] -> w475
          frame True {
            w479 = T8[] [enum."-find center", enum."-mapping"] items=["empty", "-find center", "-mapping", "fit", "-shake it one", "bbb", "-update pond", "move z(center)", "move z(inf)", "update pond", "fancy fit one", "fragment window moves", "-shake it two", "fancy fit two", "pm fit"]
          }
          frame False {
            w480 = T8[] [enum."-update pond", enum."-find center", enum."-mapping"] items=["empty", "-find center", "-mapping", "fit", "-shake it one", "bbb", "-update pond", "move z(center)", "move z(inf)", "update pond", "fancy fit one", "fragment window moves", "-shake it two", "fancy fit two", "pm fit"]
          }
        }
        n141 = call "find peak action stack.vi"("stack action"=stack_action_--_control."push", "find peak action list"=w475, "command stack"=w478) -> ("command stack out"=w476:T8[])  [unwired: 6 in, 2 out]
      }
      frame "fancy fit one" {
        n142 = Unbundle By Name(w486) -> ("wavepacket is"=w485:bool)
        n143 = case shown="False" w485 {
          tunnel: [w497 w498] -> w493
          frame True {
            w497 = T8[] [enum."-find center", enum."-mapping", enum."-shake it one"] items=["empty", "-find center", "-mapping", "fit", "-shake it one", "bbb", "-update pond", "move z(center)", "move z(inf)", "update pond", "fancy fit one", "fragment window moves", "-shake it two", "fancy fit two", "pm fit"]
          }
          frame False {
            w498 = T8[] [enum."-update pond", enum."-find center", enum."-mapping", enum."-shake it one"] items=["empty", "-find center", "-mapping", "fit", "-shake it one", "bbb", "-update pond", "move z(center)", "move z(inf)", "update pond", "fancy fit one", "fragment window moves", "-shake it two", "fancy fit two", "pm fit"]
          }
        }
        n144 = Bundle By Name(cluster=w484, "cursor bracket: fragment  ref"=w481, "fancy fit.shakeit counter"=0) -> (w482:T12)
        n145 = call "find peak action stack.vi"("stack action"=stack_action_--_control."push", "find peak action list"=w493, "command stack"=w496) -> ("command stack out"=w494:T8[])  [unwired: 6 in, 2 out]
      }
      frame "fancy fit two" {
        n146 = Unbundle By Name(w504) -> ("wavepacket is"=w503:bool)
        n147 = case shown="True" w503 {
          tunnel: [w515 w516] -> w511
          frame True {
            w515 = T8[] [enum."-find center", enum."-mapping", enum."-shake it two"] items=["empty", "-find center", "-mapping", "fit", "-shake it one", "bbb", "-update pond", "move z(center)", "move z(inf)", "update pond", "fancy fit one", "fragment window moves", "-shake it two", "fancy fit two", "pm fit"]
          }
          frame False {
            w516 = T8[] [enum."-update pond", enum."-find center", enum."-mapping", enum."-shake it two"] items=["empty", "-find center", "-mapping", "fit", "-shake it one", "bbb", "-update pond", "move z(center)", "move z(inf)", "update pond", "fancy fit one", "fragment window moves", "-shake it two", "fancy fit two", "pm fit"]
          }
        }
        n148 = Bundle By Name(cluster=w502, "cursor bracket: fragment  ref"=w499, "fancy fit.shakeit counter"=0) -> (w500:T12)
        n149 = call "find peak action stack.vi"("stack action"=stack_action_--_control."push", "find peak action list"=w511, "command stack"=w514) -> ("command stack out"=w512:T8[])  [unwired: 6 in, 2 out]
      }
      frame "-update pond" {
        n150 = Unbundle By Name(w521) -> ("number of 2D grid points"=w520:i32, "pond scale factor"=w518:dbl)
        n151 = call "find fit -- set up complex region - V2.vi"("scale factor"=w518) -> ("complex region"=w517:T7)  [unwired: 10 in]
        n152 = call "generate wave packet V2.vi"("number of grid points"=w520, "complex region"=w517, "wavepacket in"=w522) -> ("pond array out"=w524:cdb[][], "wavepacket array out"=w525:cdb[][], "wavepacket out"=w526:T4)  [unwired: 6 in]
        n153 = Bundle By Name(cluster=w526, "wavepacket is"=TRUE) -> (w523:T4)
      }
      frame "pm fit" {
        n154 = Unbundle By Name(w538) -> ("omega in window"=w537:dbl[], "z in window"=w536:cdb[])
        n155 = Unbundle By Name(w531) -> ("span"=w542:dbl)
        n156 = call "filter - complex - four.vi"("omega  in"=w537, "z in"=w536, "span"=w542) -> ("center"=w548:cdb, "norm"=w547:dbl, "omega out"=w549:dbl[], "z in out"=w550:cdb[], "z out"=w543:cdb[], "win omega out"=w546:dbl[], "dz/domega out"=w545:cdb[], "tale of three"=w551:T18)  [unwired: 9 in]
        n157 = call "peak -- PM find lorenzian - V2.vi"("omega"=w549, "z"=w543, "dz/domega"=w545) -> ("phase (around center)"=w544:dbl[], "weights"=w534:dbl[], "cp lorentzian"=w540:T1, "poor man lorentzian"=w535:T1)  [unwired: 9 in]
        "pm lorentzian" <- w535
        "cp lorentzian" <- w540
        "good lorentzian" <- w535
        n158 = case shown="\"plot cp\"" enum16{"plot pm", "plot cp", "a"}."plot pm" ("plot what") {
          tunnel: [w571 w572] -> w533
          tunnel: w540 -> [_ w572]
          tunnel: w535 -> [w571 _]
          frame "plot pm", Default {
          }
          frame "plot cp" {
          }
        }
        n159 = case shown="\"plot\", Default" w532 {
          tunnel: w551 -> [w570 _]
          tunnel: w550 -> [w569 _]
          tunnel: w549 -> [w568 _]
          tunnel: w548 -> [w567 _]
          tunnel: w547 -> [w566 _]
          tunnel: w546 -> [w565 _]
          tunnel: w544 -> [w564 _]
          tunnel: w543 -> [w563 _]
          tunnel: w539 -> [w562 _]
          tunnel: w531 -> [w561 _]
          tunnel: w534 -> [w560 _]
          tunnel: w533 -> [w559 _]
          frame "plot", Default {
            n160 = call "filter pipe - plot staff - more - V2.vi"("omega  in"=w568, "zin"=w569, "z out"=w563, "win omega"=w565, "phase"=w564, "dz/domega in"=w560, "center"=w567, "plots: filter related"=w562, "norm"=w566, "parameters: complex fit"=w561, "tale of three indices -- int -- control"=w570, "lorentzian"=w559) -> ()  [unwired: 8 in]
          }
          frame "dont plot" {
          }
        }
      }
    }
    n161 = call "find peak action stack.vi"("stack action"=stack_action_--_control."check", "command stack"=w49) -> ("stack is empty ?"=w43:bool, "command stack out"=w46:T8[])  [unwired: 7 in, 1 out]
  }
  "lorentzian out" <- w13
  "single fit parameters out" <- w12
  "omega map parameters out" <- w11
  "complex region out" <- w14
  "parameters: wavepacket  out" <- w10
